vi "Edit a Button--Material.vi"() -> ()   [LabVIEW 2021, in "TSC Button Editor.lvclass"]
doc: "Edit/create buttons based on a few built-in templates.\n\n<b>Code Developed By:</b>\nTechnology Service Corporation\n1983 S Liberty Drive\nBloomington, IN 47403\nPhone: 812 558-7100\nwww.tsc.com/atcs\n\nDeveloper:\nDaniel Coons"
uses:
  TSC Button Editor.lvclass
  TSC Button Editor.lvclass/TSC Button Editor.ctl
  <vilib>/Utility/miscctls.llb/LVPositionTypeDef.ctl
  user32.dll
  Material Theme/Material Theme.lvclass
  Material-Scheme/Material-Scheme.lvclass
panel:
  in  "Tab Control 2":enum32{"Button Format", "Glyphs"}(tab)
  in  "Lock Text in Center?":bool
  in  "update text format":bool
  in  "Boolean Colors":T1={"false color"={"border"=15922170, "fill"=15922170}, "true color"={"border"=14936305, "fill"=14936305}, "click false color"={"border"=14410221, "fill"=14410221}, "click true color"={"border"=14410221, "fill"=14410221}, "hover false color"={"border"=14540516, "fill"=14540516}, "hover true color"={"border"=14540516, "fill"=14540516}}
  in  "Boolean Text Format":T2={"Font:Color"=3563918, "Font:Bold?"=TRUE, "Font:Name"="App Font", "Font:Size"=22}
  in  "Boolean Text":string
  in  "update colors":bool
  in  "Button Size":cluster{"Width":u32, "Height":u32}={"Width"=204, "Height"=48}
  in  "update button size":bool
  in  "Button Text Location":cluster{"Left":i32, "Top":i32}
  in  "update button text location":bool
  in  "edit":bool
  out "Images":T3(array[cluster]) caption="Array"
  in  "Filter":string
  out "images directory":path
  in  "Button Family":u16(ring) items=["(1) Small Button Single Image 24px", "(2) Small Button Text Only", "(3) Large Button Single Image 40px", "(4) Large Button Text Only", "(5) Small Button Multi Image 24px", "(6) Large Button Multi Image 40px", "(7) Floating Action Button (FAB)"]
  in  "Color Level":u16(ring) items=["Primary", "Secondary", "Tertiary", "Error", "Primary Fixed", "Secondary Fixed", "Tertiary Fixed"]
  in  "Theme":u16(ring) items=["Light Theme", "Light Medium Contrast", "Light High Contrast", "Dark Theme", "Dark Medium Contrast", "Dark High Constrast"]
  in  "theme path":path
  in  "Open":bool
  in  "Button Type":u16(ring) items=["elevated--rectangular--icon.ctl", "elevated--rounded--icon.ctl", "filled--rectangular--icon.ctl", "filled--rounded--icon.ctl", "nooutline--rectangular--icon.ctl", "nooutline--rounded--icon.ctl", "outline--rectangular--icon.ctl", "outline--rounded--icon.ctl", "tonal--rectangular--icon.ctl", "tonal--rounded--icon.ctl", "transparent--rectangular--icon.ctl", "transparent--rounded--icon.ctl"]
  in  "Tab Control":enum32{"Button Formatting"}(tab)
  in  "Image Color":u32(colorbox)=3563918
  in  "Button Image":path
  in  "Button Images":T4
  in  "Multiple Colors":T5={"False Color"=3563918, "True Color"=3563918, "True Press"=3563918, "False Press"=3563918}
  out "b":u8
  out "g":u8
  out "r":u8
  out "Color":u32(colorbox)
  in  "Hex Color":u32 max=16777215 format="%06x"
  in  "close":bool
  out "header":bool
  in  "Save":bool
  out "error out":errorcluster
  # "Note: match the size of the replacement image so scaling is correct.\nNormal size: 24x24px, Large size: 40x40px, Icon size: 30x30px\n\nFor other desired sizes, save the control and open it in LabVIEW. Click the Wrench in the tool bar to change to Edit Mode."
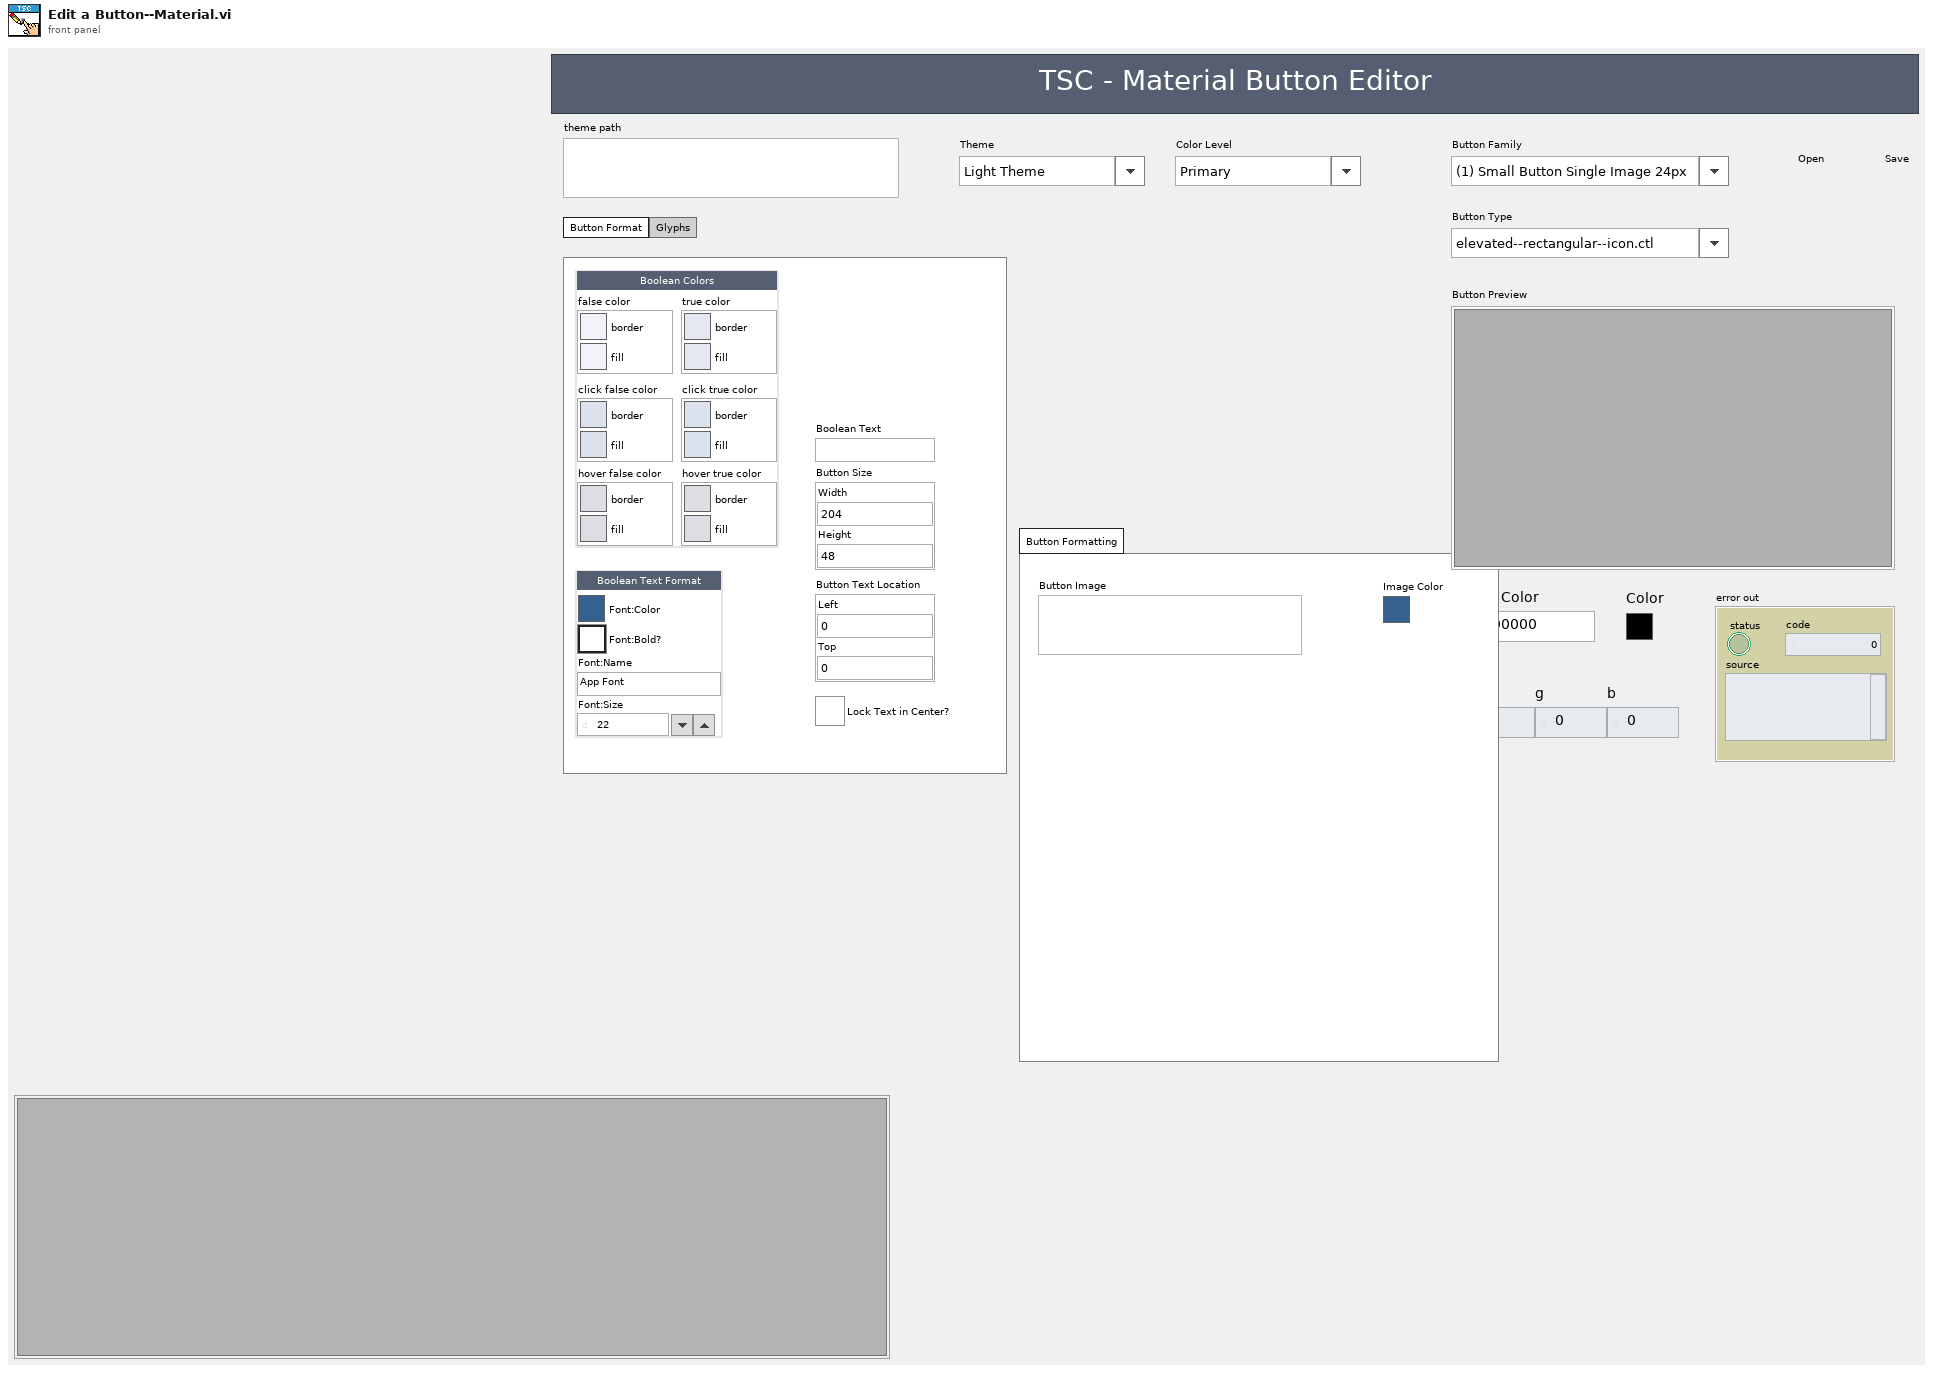
[diagram p1: front panel]
types:
  T1 = cluster{"false color":cluster{"border":u32, "fill":u32}, "true color":cluster{"border":u32, "fill":u32}, "click false color":cluster{"border":u32, "fill":u32}, "click true color":cluster{"border":u32, "fill":u32}, "hover false color":cluster{"border":u32, "fill":u32}, "hover true color":cluster{"border":u32, "fill":u32}}
  T2 = cluster{"Font:Color":u32, "Font:Bold?":bool, "Font:Name":string, "Font:Size":u32}
  T3 = cluster{"2D Picture":picture, "path":path, "image-name":string}[][]
  T4 = cluster{"False Image":path, "True Image":path, "True Press":path, "False Press":path}
  T5 = cluster{"False Color":u32, "True Color":u32, "True Press":u32, "False Press":u32}
  T6 = cluster{"2D Picture":picture, "path":path, "image-name":string}[]
  T7 = typedef "TSC Button Editor.lvclass/User Events.ctl" = cluster{"update colors":refnum<user-event>, "update boolean data":refnum<user-event>, "update image":refnum<user-event>, "update multi image":refnum<user-event>}
  T8 = typedef "LVPositionTypeDef.ctl" = cluster{"Left":i32, "Top":i32}
  T9 = enum32{"invalid VI type", "Standard VI", "Control VI", "Global VI", "Polymorphic VI", "Configuration VI", "SubSystem", "Facade VI", "Method VI", "Statechart Diagram VI"}
  T10 = typedef "LVBoundsTypeDef.ctl" = cluster{"Width":u32, "Height":u32}
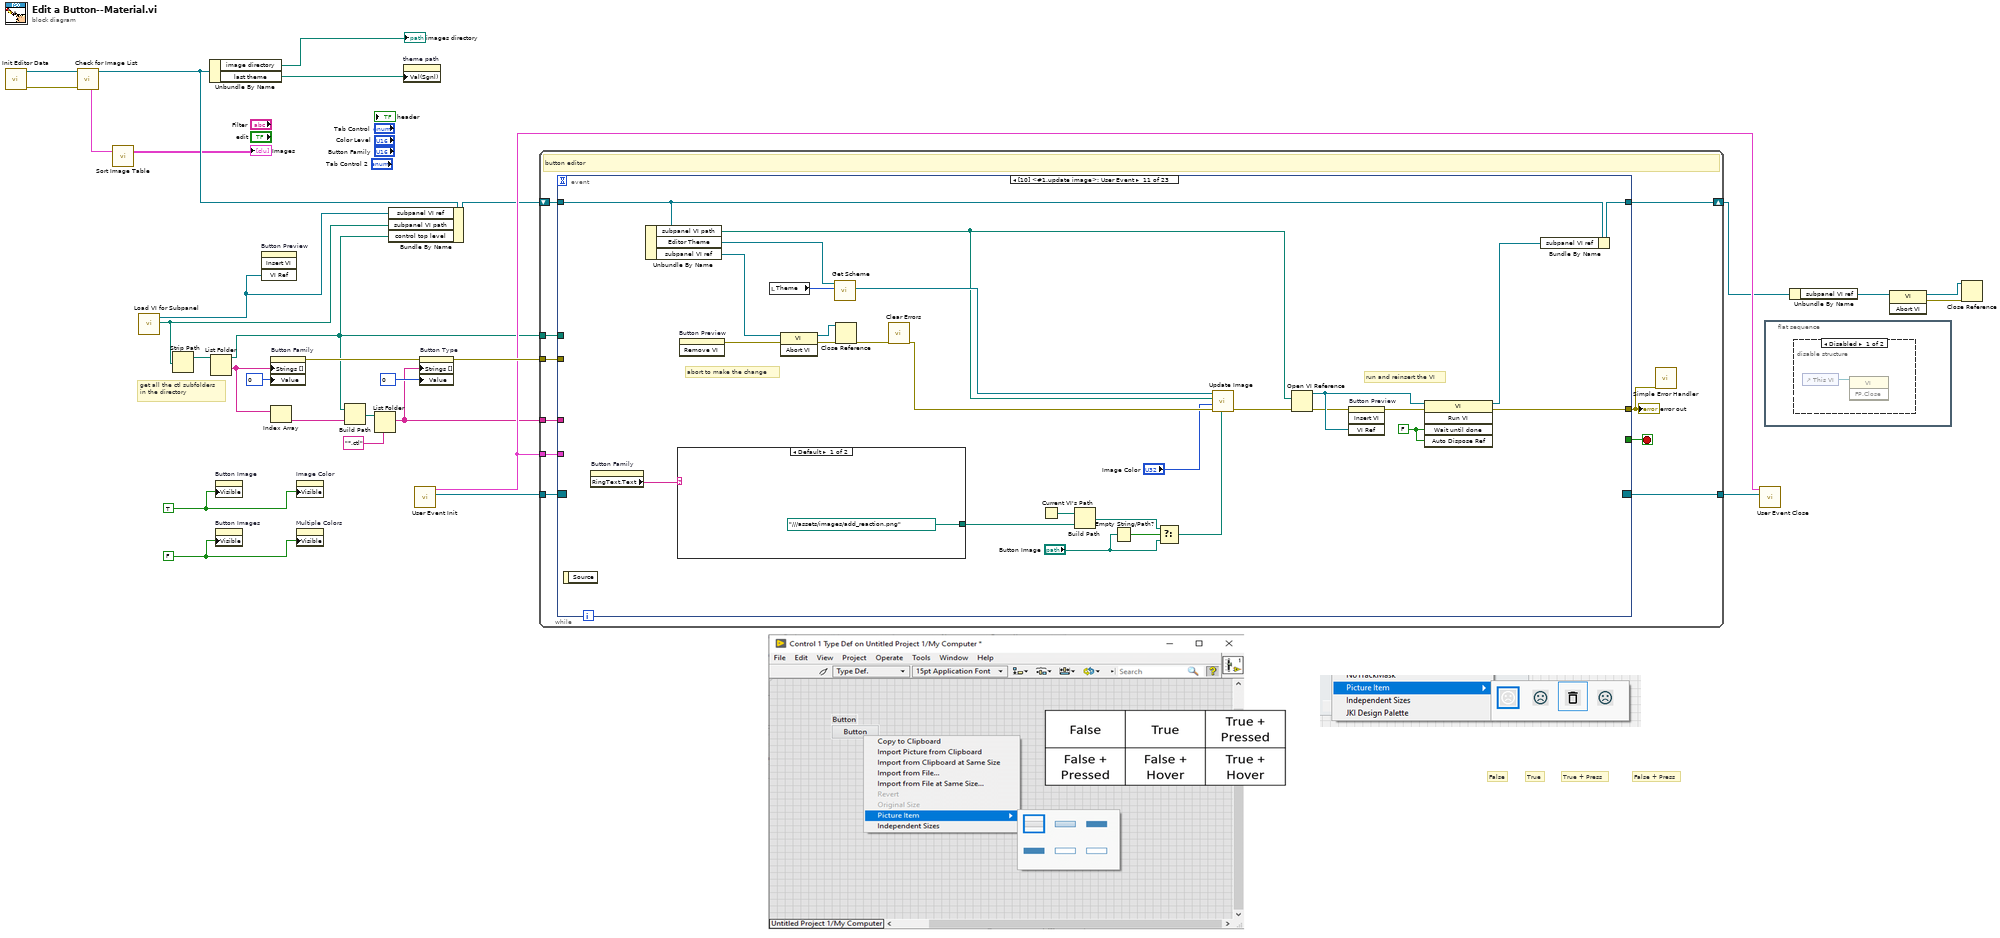
[diagram p0: block diagram]
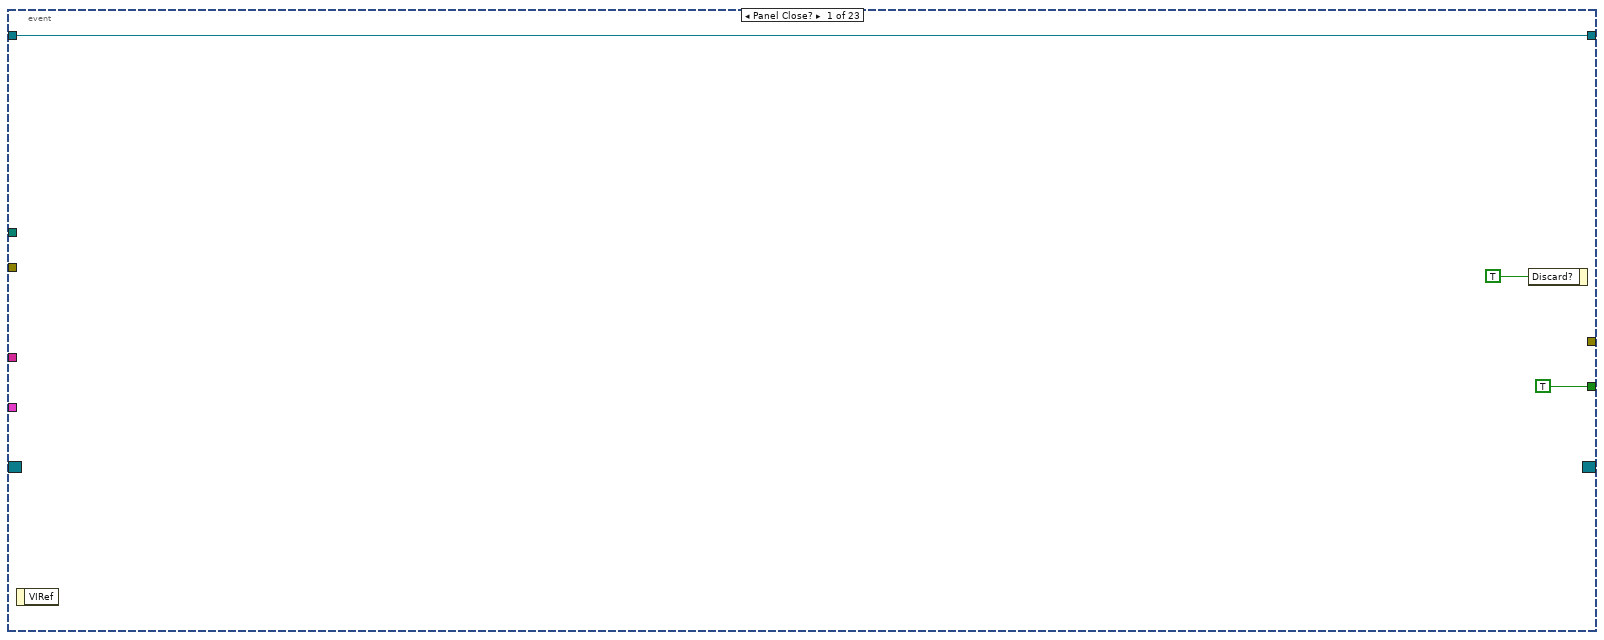
[diagram p3: hidden frame]
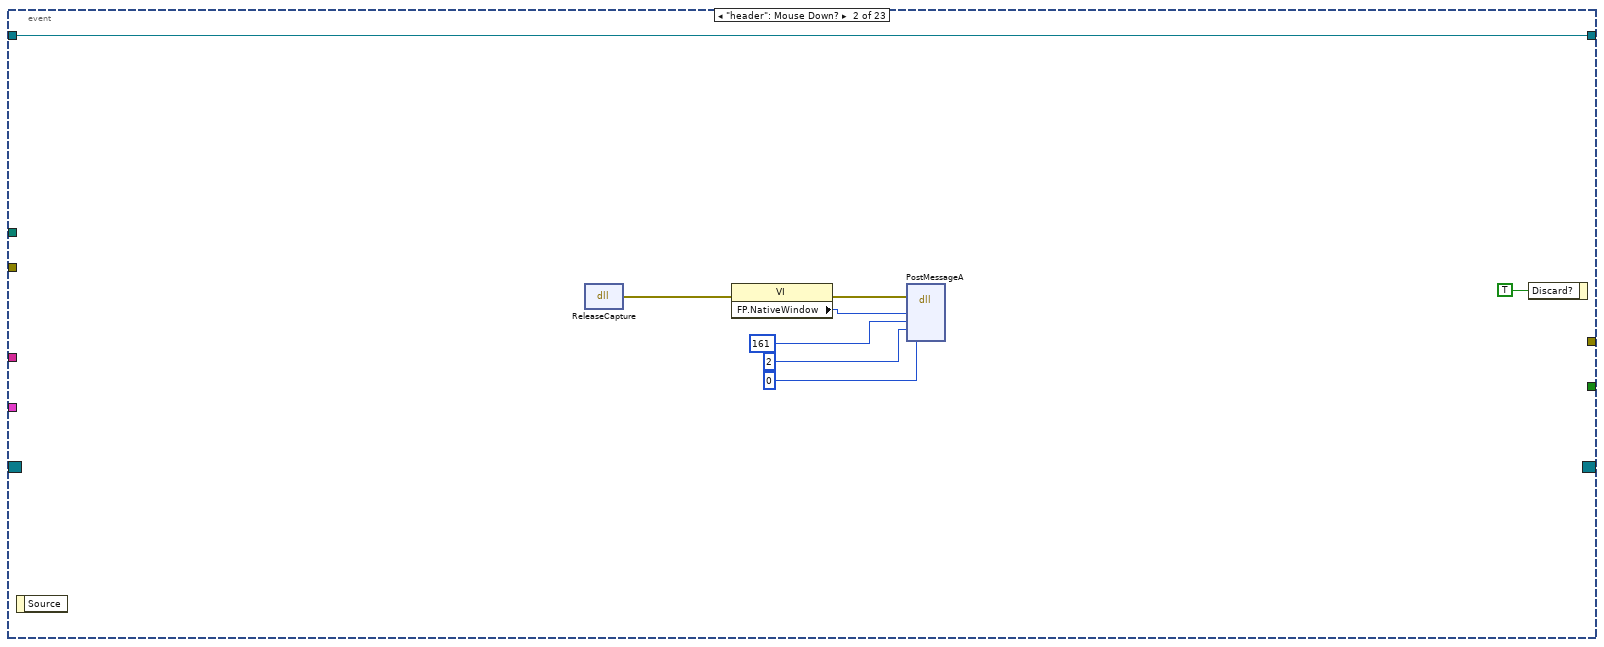
[diagram p4: hidden frame]
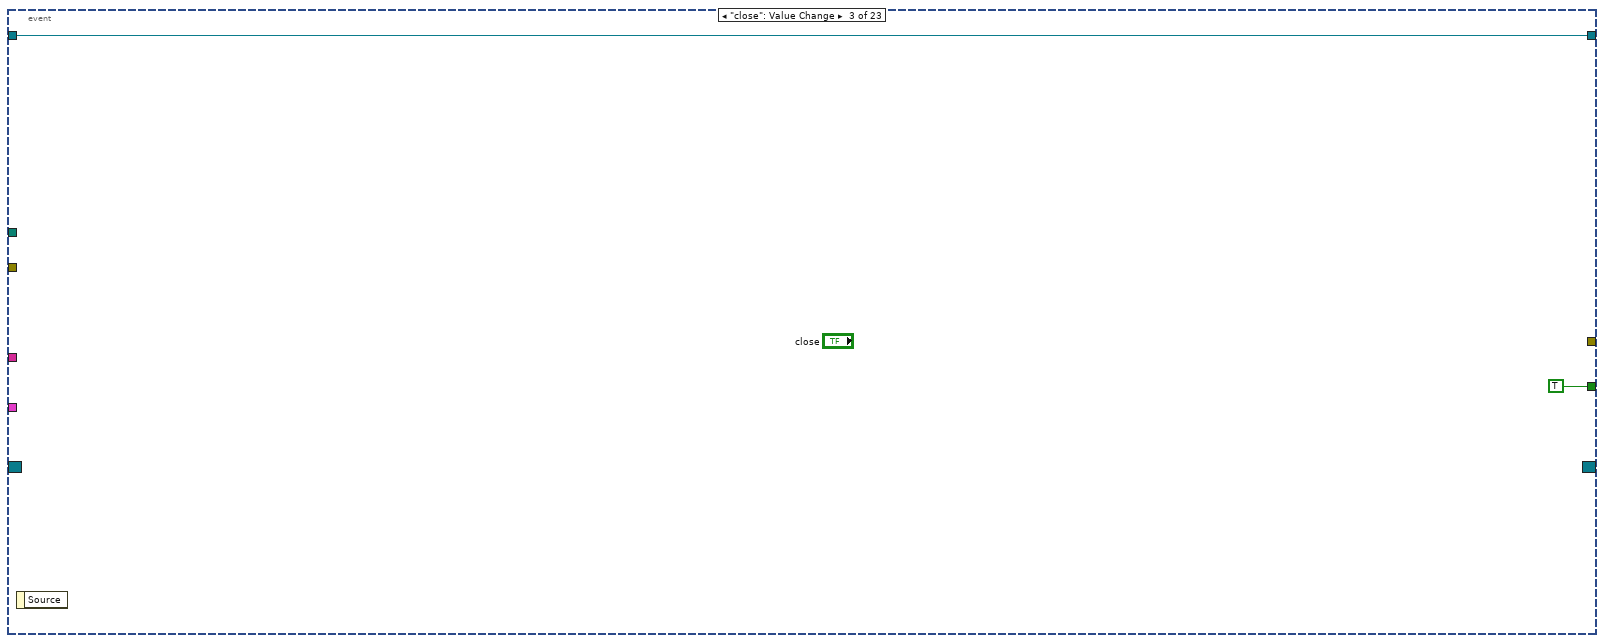
[diagram p5: hidden frame]
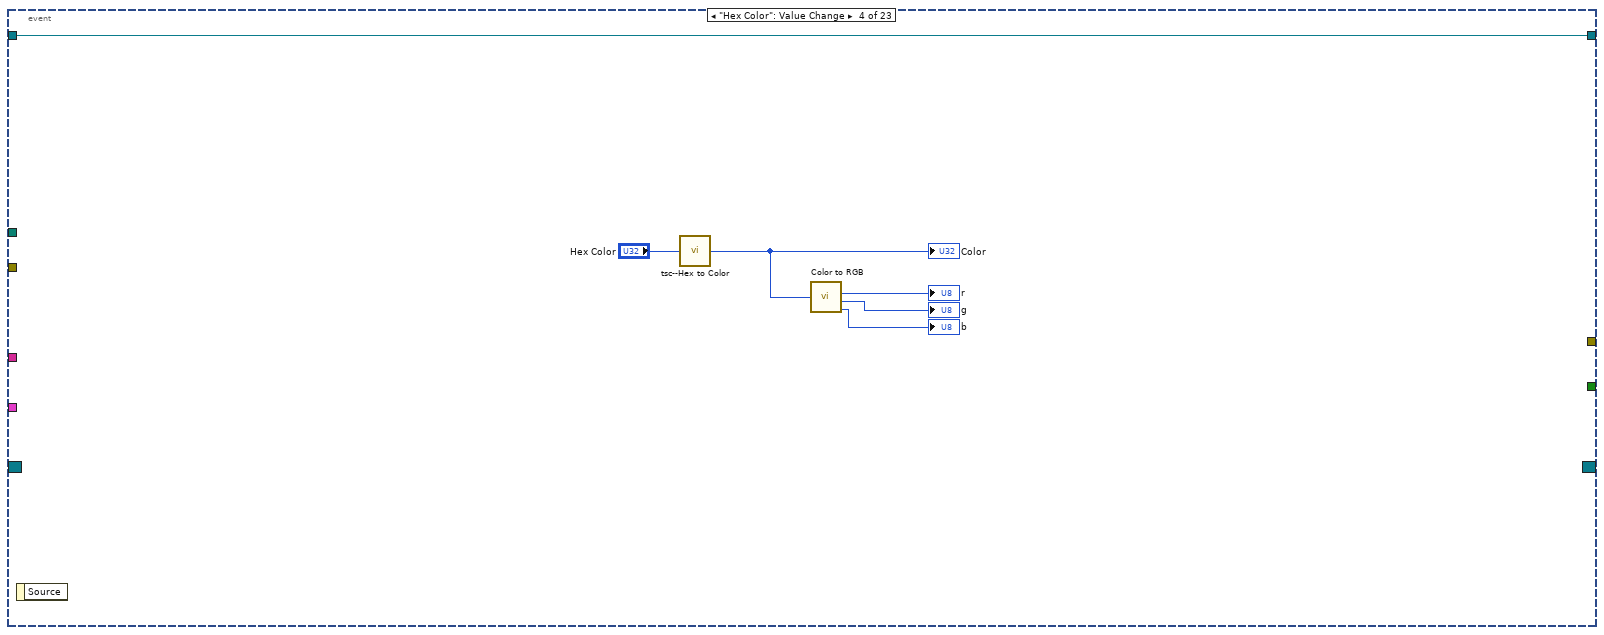
[diagram p6: hidden frame]
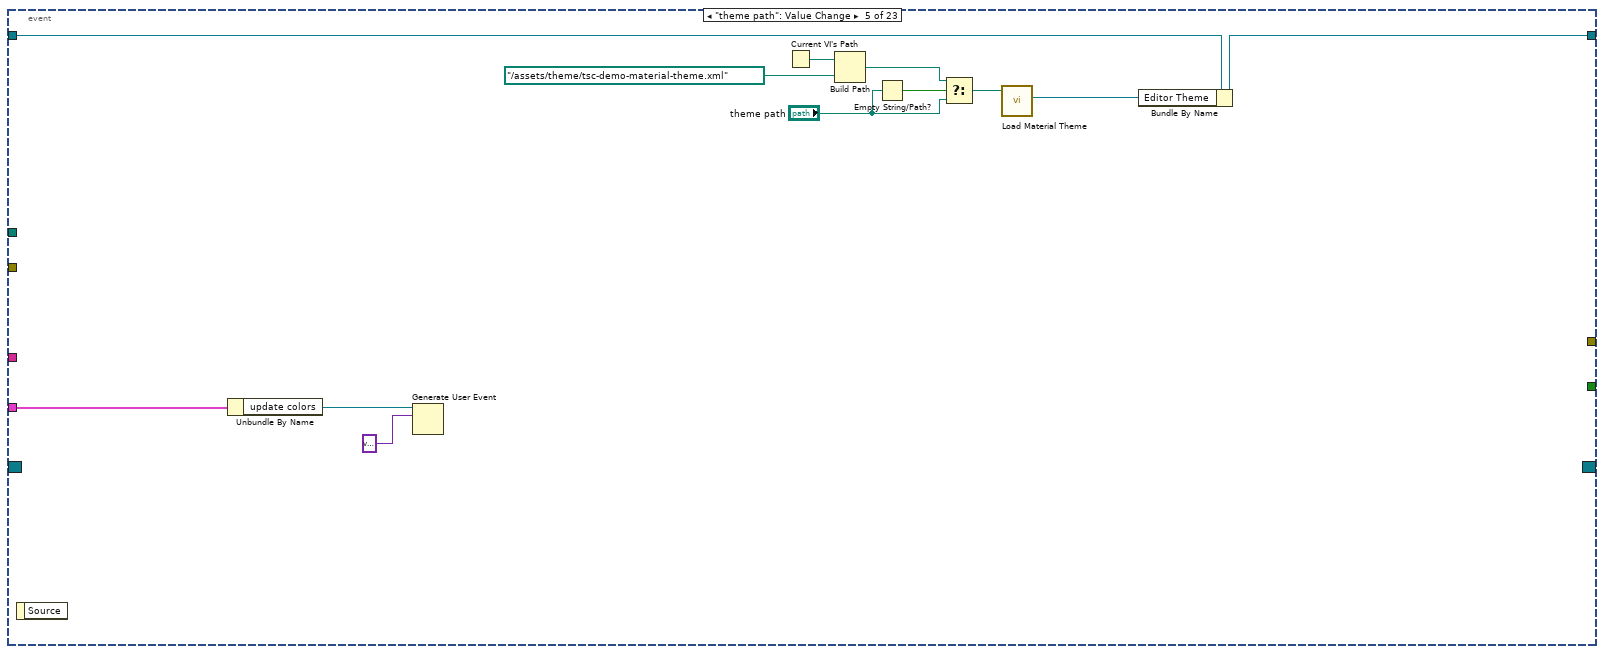
[diagram p7: hidden frame]
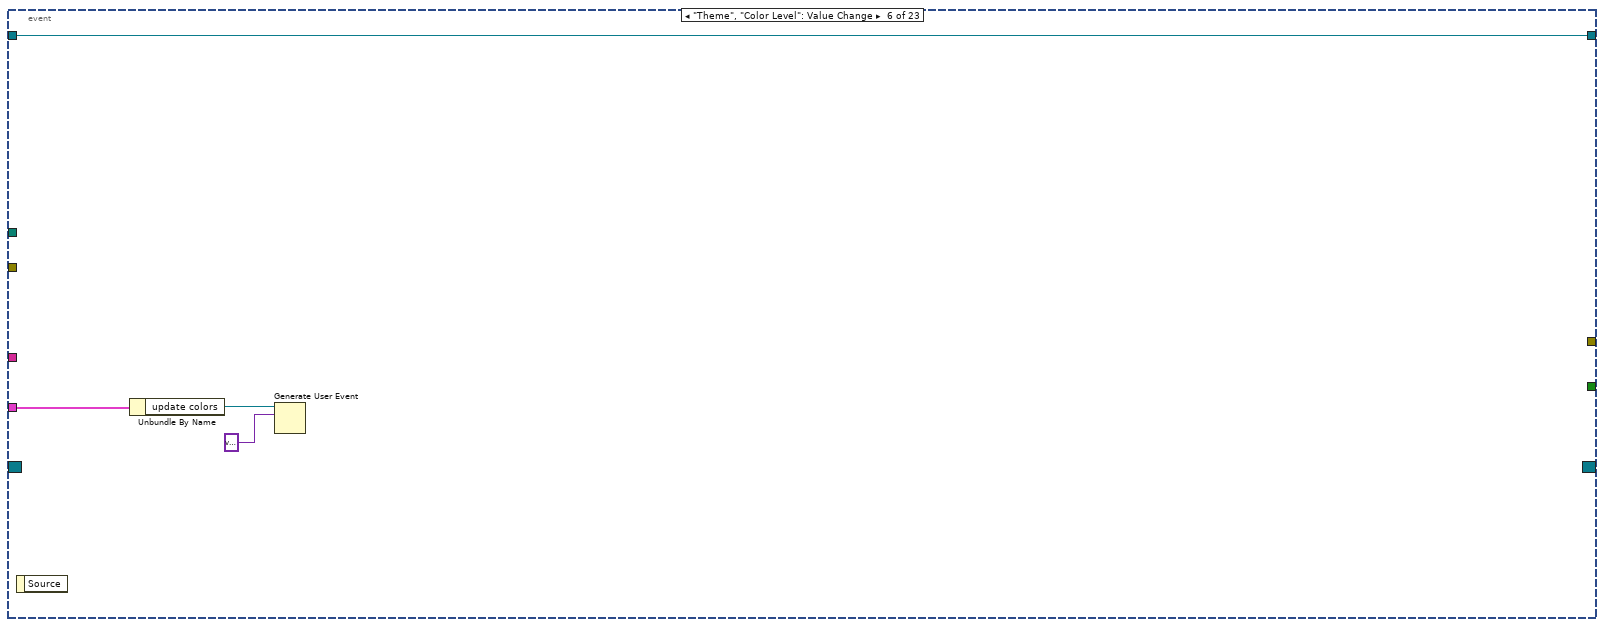
[diagram p8: hidden frame]
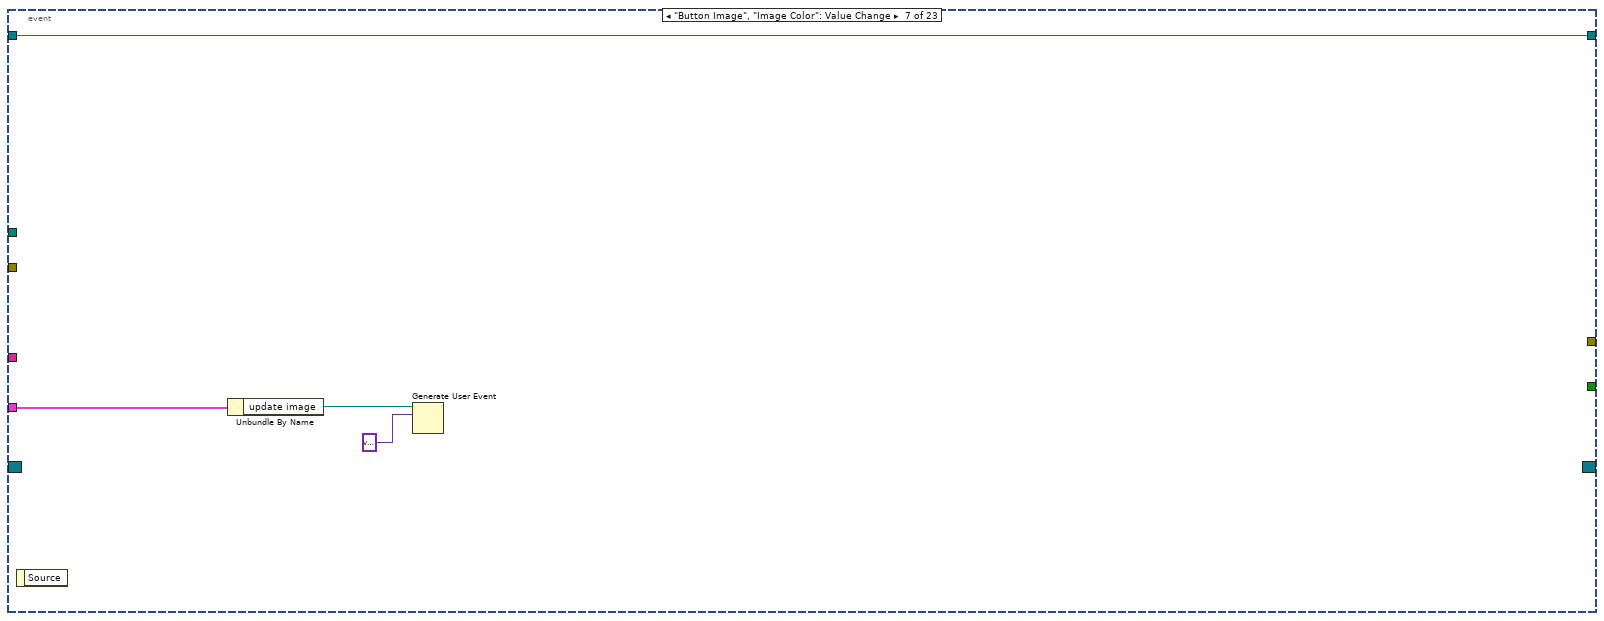
[diagram p9: hidden frame]
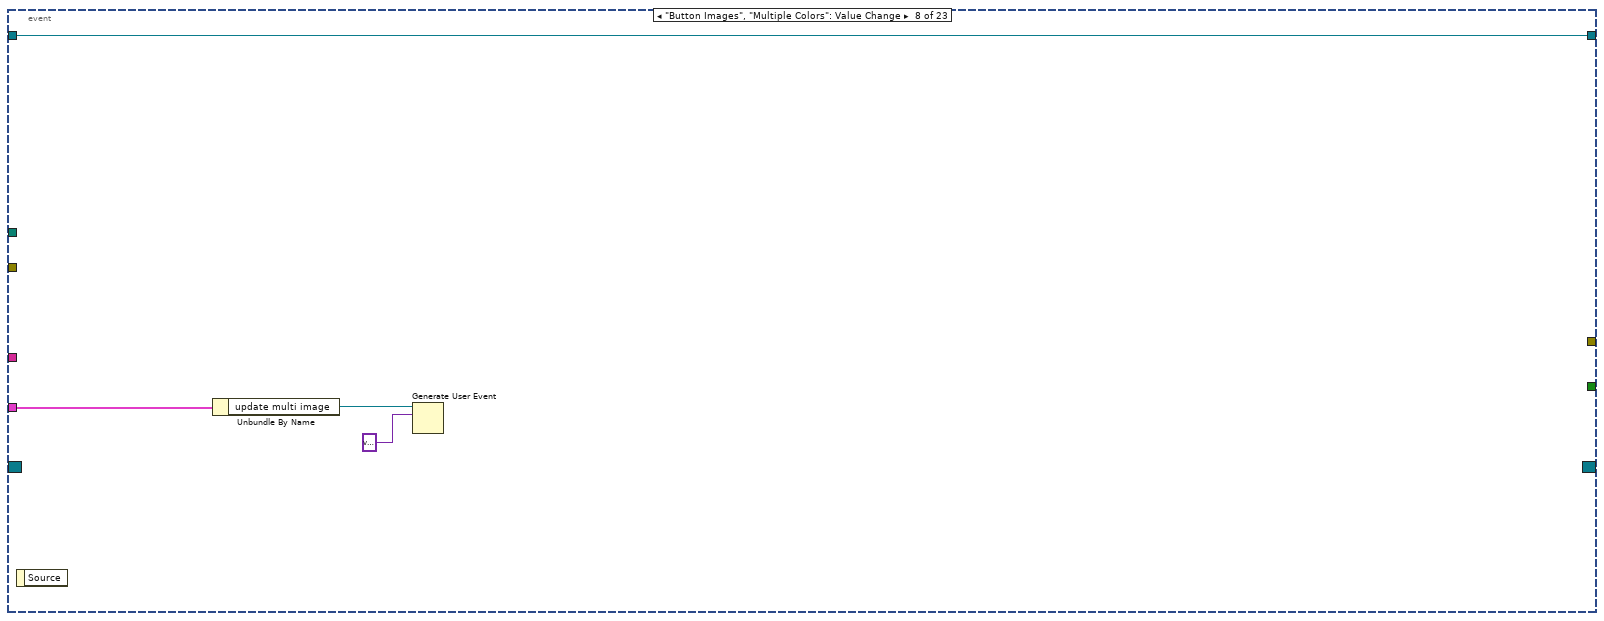
[diagram p10: hidden frame]
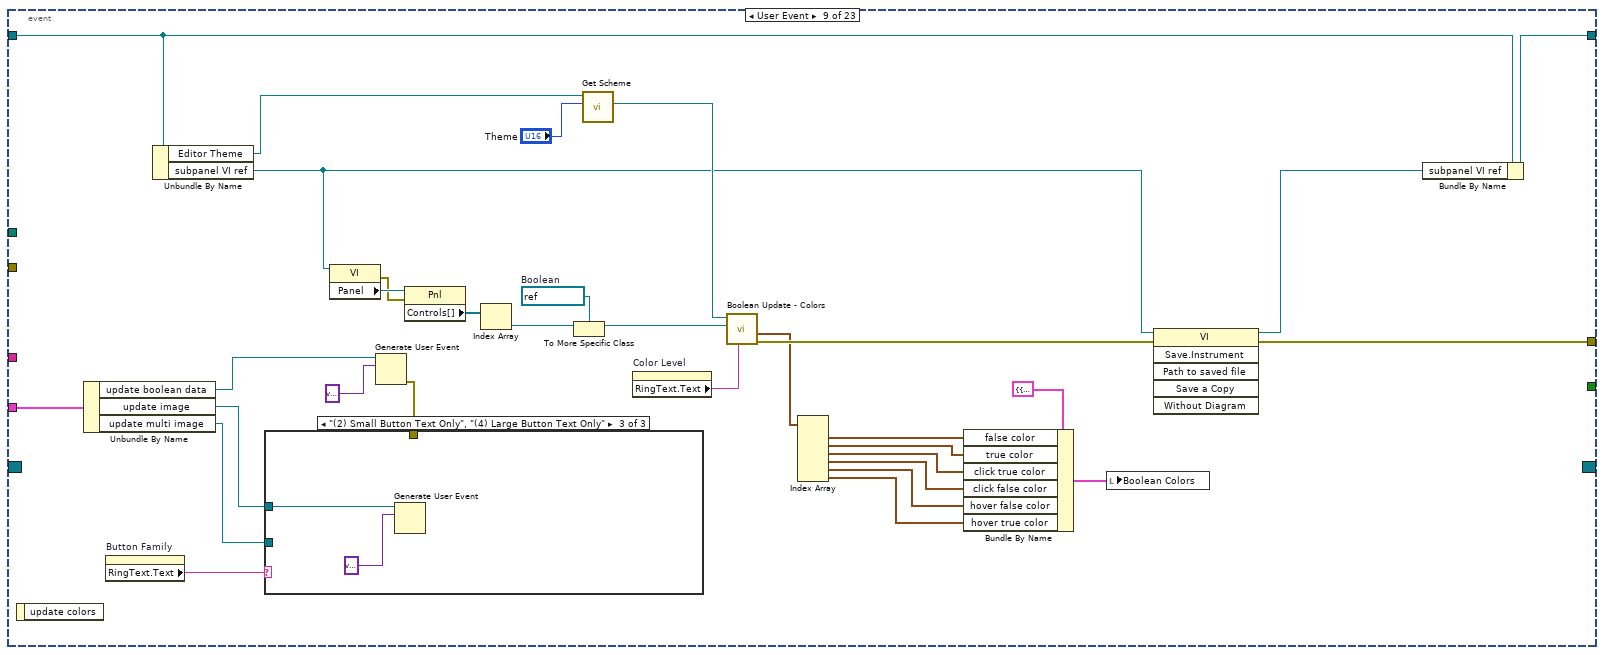
[diagram p11: hidden frame]
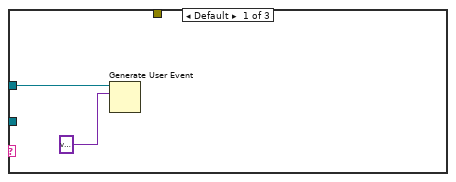
[diagram p12: hidden frame]
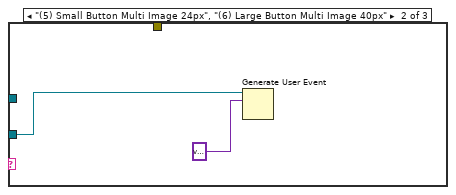
[diagram p13: hidden frame]
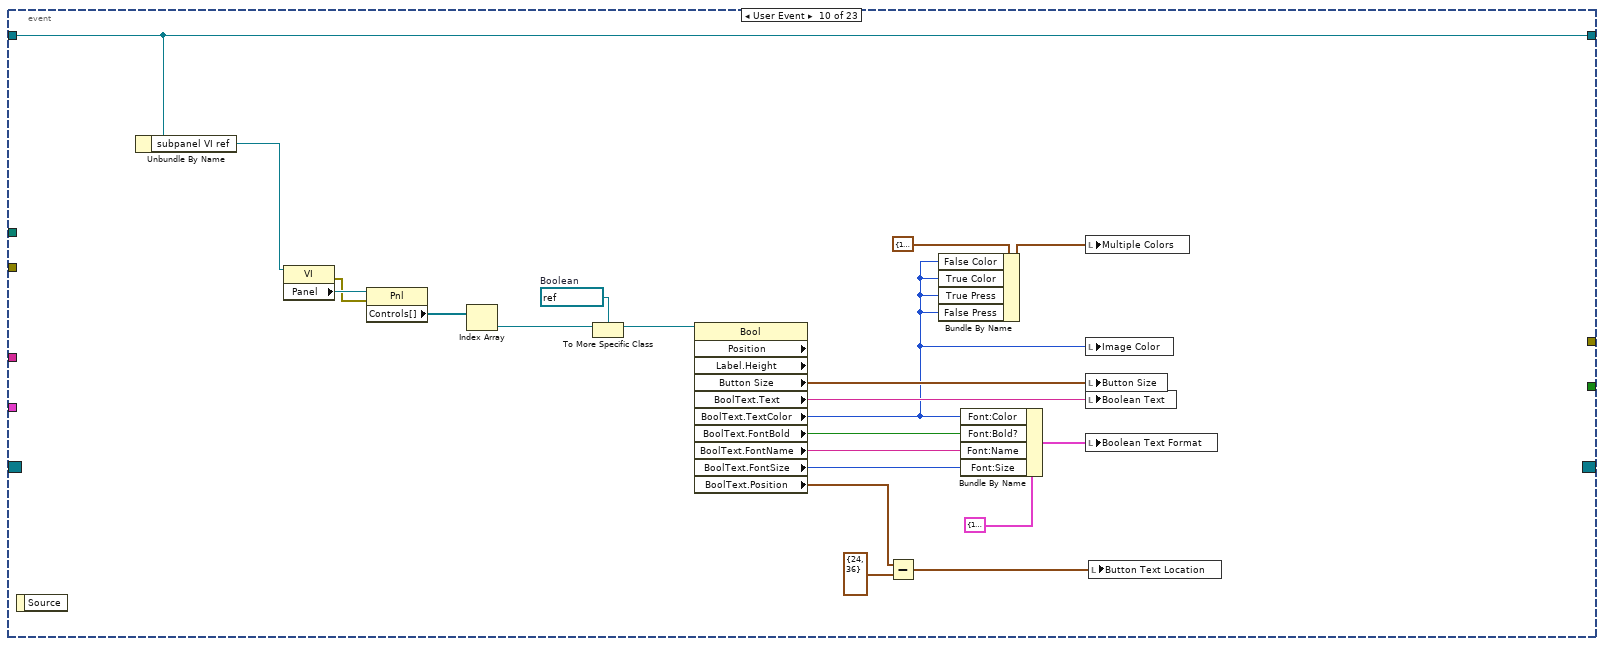
[diagram p14: hidden frame]
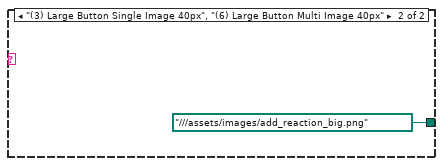
[diagram p15: hidden frame]
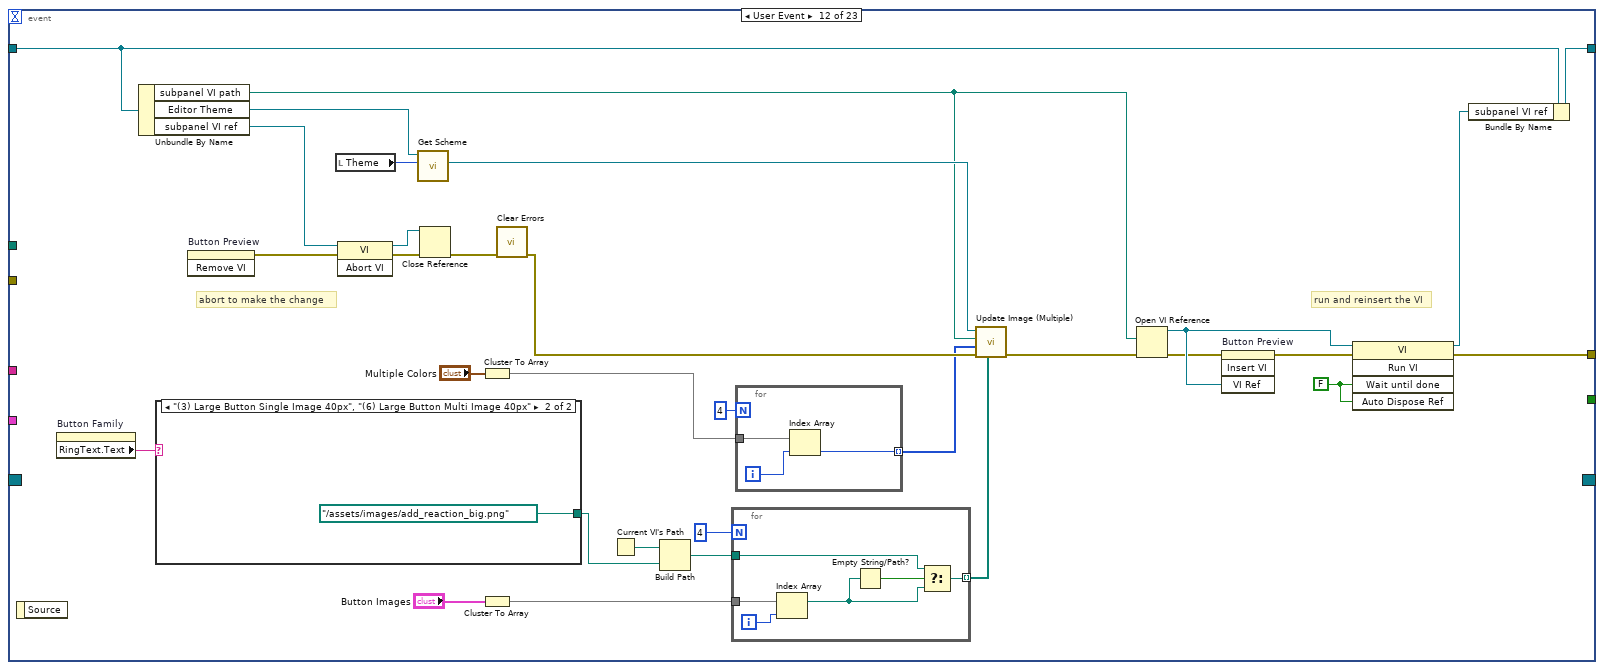
[diagram p16: hidden frame]
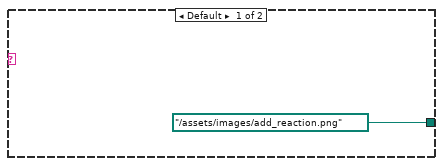
[diagram p17: hidden frame]
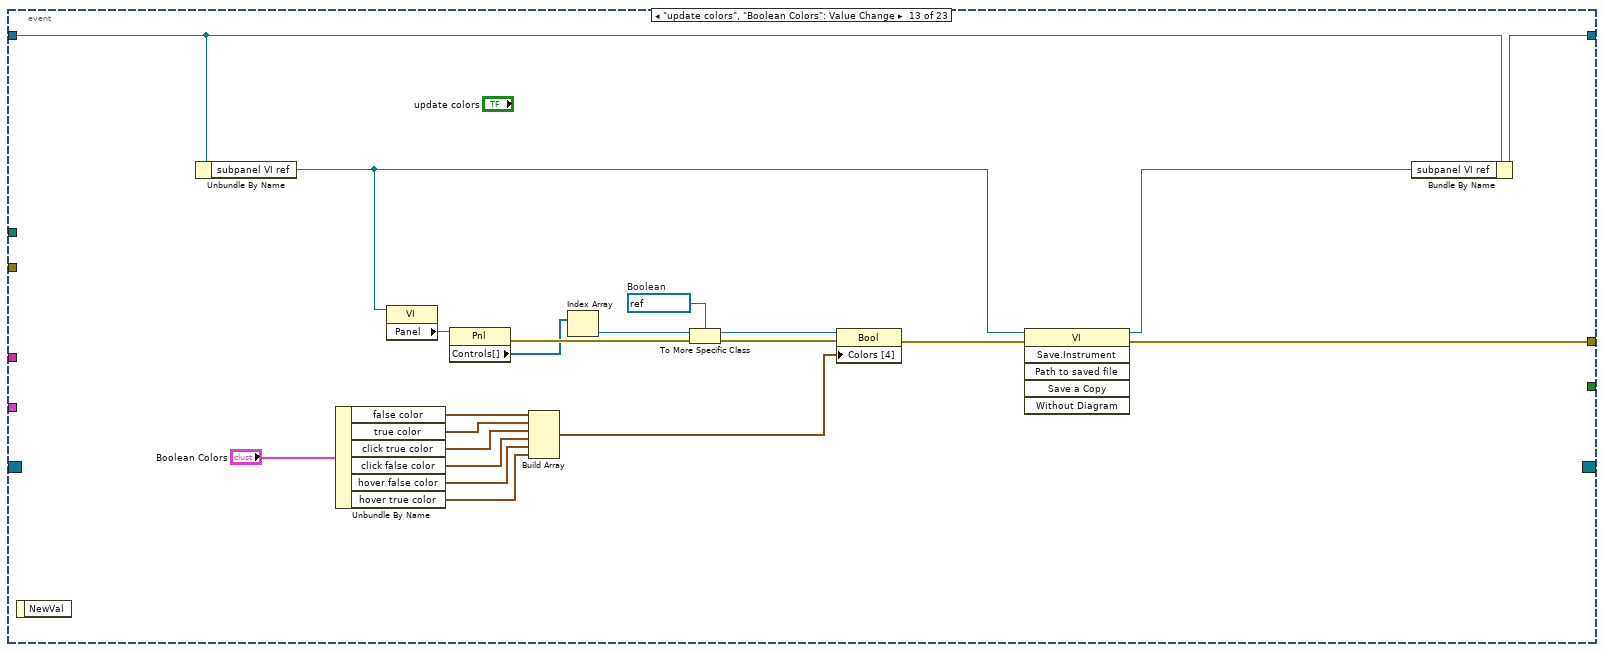
[diagram p18: hidden frame]
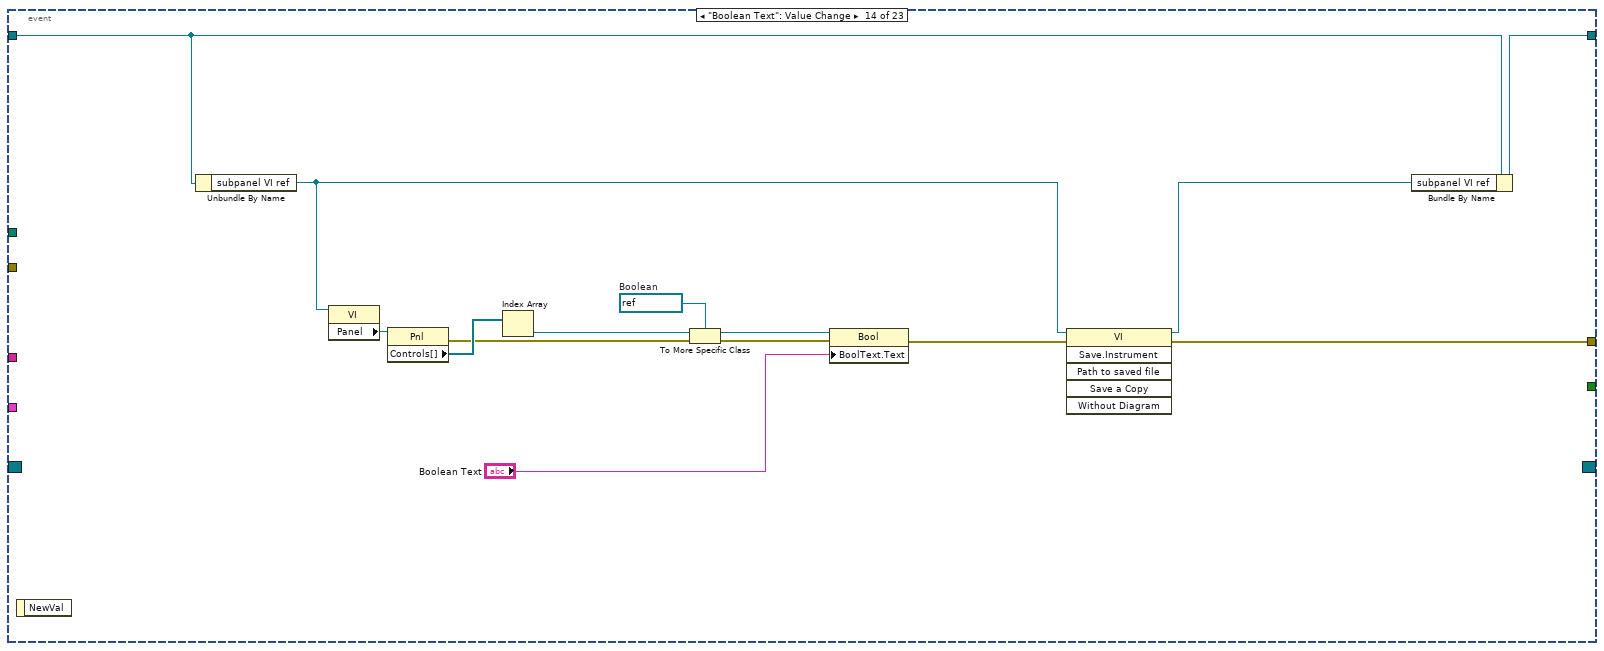
[diagram p19: hidden frame]
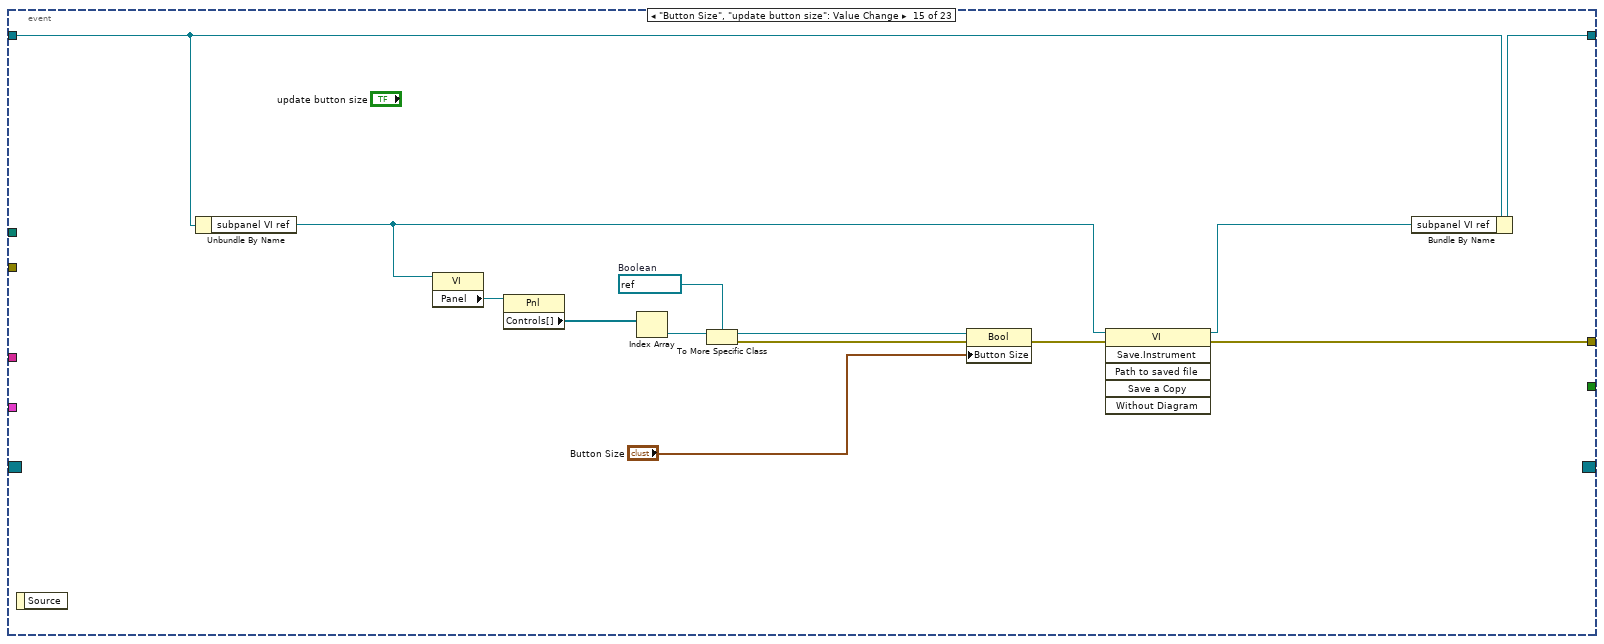
[diagram p20: hidden frame]
diagram:
  w14 = FALSE
  w15 = TRUE
  w17 = u16 0 items=[""] ("Button Type")
  w22 = u16 0 items=[""] ("Button Family")
  # "False + Press"
  # "True + Press"
  # "True"
  # "False"
  # "get all the ctl subfolders\nin the directory"
  n1 = call "Init Editor Data.vi"() -> ("error out"=w1:errorcluster, "TSC Button Editor"=w5:refnum<class "TSC Button Editor.lvclass">)  [unwired: 10 in]
  n2 = call "Check for Image List.vi"("error in"=w1, "TSC Button Editor in"=w5) -> ("TSC Button Editor out"=w4:refnum<class "TSC Button Editor.lvclass">, "Images"=w3:T6)  [unwired: 7 in, 1 out]
  n3 = call "Sort Image Table.vi"("Images in"=w3) -> ("Images out"=→"Images":T3)  [unwired: 2 in]
  n4 = call "Load VI for Subpanel.vi"() -> ("VI Path"=w9:path, "VI out"=w10:refnum<vi>)  [unwired: 10 in]
  n5 = Strip Path(path=w9) -> (stripped path=w27:path)  [unwired: 1 out]
  n6 = Unbundle By Name(w4) -> ("image directory"=→"images directory":path, "last theme"=w13:path)
  n7 = List Folder(path=w27) -> (path out=w8:path, folder names=w21:string[])  [unwired: 3 in, 2 out]
  n8 = property on="Button Image" class="Path"("Visible"=w15) -> ()  [unwired: 2 in, 2 out]
  n9 = property on="Button Images" class="Clust (strict)"("Visible"=w14) -> ()  [unwired: 2 in, 2 out]
  n10 = invoke on="Button Preview" class="SubPnl" method="Insert VI"("VI Ref"=w10) -> ()  [unwired: 3 in, 4 out]
  n11 = property on="Button Family" class="Ring (strict)"("Strings []"=w21, "Value"=w22) -> (error out=w23:errorcluster)  [unwired: 2 in, 1 out]
  n12 = Index Array(array=w21) -> (element=w20:string)  [unwired: 1 in]
  n13 = property on="Image Color" class="ColBox"("Visible"=w15) -> ()  [unwired: 2 in, 2 out]
  n14 = property on="Multiple Colors" class="Clust (strict)"("Visible"=w14) -> ()  [unwired: 2 in, 2 out]
  n15 = Build Path(base path=w8, name or relative path=w20) -> (appended path=w19:path)
  n16 = List Folder(path=w19, pattern="*.ctl") -> (filenames=w16:string[])  [unwired: 2 in, 3 out]
  n17 = Bundle By Name(cluster=w4, "subpanel VI ref"=w10, "subpanel VI path"=w9, "control top level"=w8) -> (w11:refnum<class "TSC Button Editor.lvclass">)
  n18 = property on="theme path" class="Path"("Val(Sgnl)"=w13) -> ()  [unwired: 2 in, 2 out]
  n19 = call "User Event Init.vi"() -> ("Event Registration Refnum"=w26:refnum<event-registration>, "user events"=w24:T7)  [unwired: 10 in]
  n20 = property on="Button Type" class="Ring (strict)"(error in=w23, "Strings []"=w16, "Value"=w17) -> (error out=w28:errorcluster)  [unwired: 1 in, 1 out]
  n21 = while {
    tunnel: w28 -> [w39]
    tunnel: w26 -> [w38]
    tunnel: [w37] -> w25
    tunnel: w24 -> [w36]
    tunnel: w16 -> [w35]
    tunnel: w8 -> [w33]
    shift-right: [w31] -> w7
    shift-left: w11 -> [w32]
    stop <- w40 stop-if-true
    # "button editor"
    n22 = event shown="[10] <#1.update image>: User Event" {
      selector: w38 -> [_ _ _ _ _ _ _ _ _ _ _ _ _ _ _ _ _ _ _ _ _ _ _]
      dyn-events: [_ _ _ _ _ _ _ _ _ _ _ _ _ _ _ _ _ _ _ _ _ _ _] -> w37
      timeout: _ -> [_ _ _ _ _ _ _ _ _ _ _ _ _ _ _ _ _ _ _ _ _ _ _]
      tunnel: [TRUE _ TRUE _ _ _ _ _ _ _ _ _ _ _ _ _ _ _ _ _ _ _ _] -> w40
      tunnel: [_ _ _ _ _ _ _ _ w110 _ w156 w190 w231 w243 w253 w262 w279 w294 w314 w344 w401 _ w430] -> w34
      tunnel: w39 -> [_ _ _ _ _ _ _ _ _ _ _ _ _ _ _ _ _ _ _ _ _ _ _]
      tunnel: w36 -> [_ _ _ _ w71 w75 w79 w83 w111 _ _ _ _ _ _ _ _ _ _ _ w390 _ _]
      tunnel: w35 -> [_ _ _ _ _ _ _ _ _ _ _ _ _ _ _ _ _ _ _ _ _ _ _]
      tunnel: w33 -> [_ _ _ _ _ _ _ _ _ _ _ _ _ _ _ _ _ _ _ _ _ _ _]
      tunnel: w32 -> [w41 w44 w52 w54 w62 w72 w76 w80 w88 w123 w145 w174 w217 w236 w250 w265 w277 w292 w310 w342 w380 w414 w428]
      tunnel: [w41 w44 w52 w54 w61 w72 w76 w80 w86 w123 w144 w173 w216 w235 w249 w264 w278 w293 w310 w342 w379 w414 w428] -> w31
      event Panel Close? {
        n23 = event-data() -> ()  [unwired: 1 in, 1 out]
        n24 = event-data("Discard?"=TRUE) -> ()  [unwired: 1 in, 1 out]
      }
      event "header": Mouse Down? {
        n25 = event-data() -> ()  [unwired: 1 in, 1 out]
        n26 = dll-call lib="user32.dll" fn="ReleaseCapture"() -> (error out=w47:errorcluster)  [unwired: 4 in, 1 out]
        n27 = property class="VI"(error in=w47) -> (error out=w46:errorcluster, "FP.NativeWindow"=w45:u64)  [unwired: 1 in, 1 out]
        n28 = dll-call lib="user32.dll" fn="PostMessageA"(error in=w46, "hWnd"=w45, "Msg"=161, "wParam"=2, "lParam"=0) -> ()  [unwired: 7 in, 2 out]
        n29 = event-data("Discard?"=TRUE) -> ()  [unwired: 1 in, 1 out]
      }
      event "close": Value Change {
        n30 = event-data() -> ()  [unwired: 1 in, 1 out]
      }
      event "Hex Color": Value Change {
        n31 = event-data() -> ()  [unwired: 1 in, 1 out]
        n32 = call "tsc--Hex to Color.vi"("Hex String"="Hex Color") -> ("Color Box"=w55:u32)  [unwired: 4 in]
        "Color" <- w55
        n33 = call <vilib>:"Color to RGB.vi"("Color"=w55) -> ("R"=→"r":u8, "G"=→"g":u8, "B"=→"b":u8)  [unwired: 1 out]
      }
      event "theme path": Value Change {
        n34 = event-data() -> ()  [unwired: 1 in, 1 out]
        n35 = Unbundle By Name(w71) -> ("update colors"=w69:refnum<user-event>)
        n36 = Generate User Event(user event=w69, event data cluster=variant ("event data")) -> ()  [unwired: 2 in, 2 out]
        n37 = Current VI's Path() -> (path=w67:path)
        n38 = Build Path(base path=w67, name or relative path=path "../assets/theme/tsc-demo-material-theme.xml") -> (appended path=w65:path)
        n39 = Empty String/Path?(string/path="theme path") -> (empty?=w68:bool)
        n40 = Select(t=w65, s=w68, f="theme path") -> (s? t:f=w63:path)
        n41 = call "Load Material Theme.vi"("file path (use dialog)"=w63) -> ("Theme"=w60:refnum<class "Material Theme.lvclass">)  [unwired: 9 in, 1 out]
        n42 = Bundle By Name(cluster=w62, "Editor Theme"=w60) -> (w61:refnum<class "TSC Button Editor.lvclass">)
      }
      event "Theme", "Color Level": Value Change {
        n43 = event-data() -> ()  [unwired: 1 in, 1 out]
        n44 = Unbundle By Name(w75) -> ("update colors"=w73:refnum<user-event>)
        n45 = Generate User Event(user event=w73, event data cluster=variant ("event data")) -> ()  [unwired: 2 in, 2 out]
      }
      event "Button Image", "Image Color": Value Change {
        n46 = event-data() -> ()  [unwired: 1 in, 1 out]
        n47 = Unbundle By Name(w79) -> ("update image"=w77:refnum<user-event>)
        n48 = Generate User Event(user event=w77, event data cluster=variant ("event data")) -> ()  [unwired: 2 in, 2 out]
      }
      event "Button Images", "Multiple Colors": Value Change {
        n49 = event-data() -> ()  [unwired: 1 in, 1 out]
        n50 = Unbundle By Name(w83) -> ("update multi image"=w81:refnum<user-event>)
        n51 = Generate User Event(user event=w81, event data cluster=variant ("event data")) -> ()  [unwired: 2 in, 2 out]
      }
      event User Event {
        w100 = refnum<vi> refnum  # Boolean
        n52 = event-data() -> ()  [unwired: 1 in, 1 out]
        n53 = Unbundle By Name(w111) -> ("update boolean data"=w113:refnum<user-event>, "update image"=w107:refnum<user-event>, "update multi image"=w108:refnum<user-event>)
        n54 = property on="Button Family" class="Ring (strict)"() -> ("RingText.Text"=w109:string)  [unwired: 2 in, 2 out]
        n55 = Unbundle By Name(w88) -> ("Editor Theme"=w84:refnum<class "Material Theme.lvclass">, "subpanel VI ref"=w87:refnum<vi>)
        n56 = property class="VI"(reference=w87) -> (error out=w102:errorcluster, "Panel"=w105:refnum<vi>)  [unwired: 1 in, 1 out]
        n57 = Generate User Event(user event=w113, event data cluster=variant ("event data")) -> (error out=w106:errorcluster)  [unwired: 2 in, 1 out]
        n58 = case shown="\"(2) Small Button Text Only\", \"(4) Large Button Text Only\"" w109 {
          tunnel: w108 -> [_ w118 _]
          tunnel: w107 -> [w116 _ w120]
          tunnel: w106 -> [_ _ _]
          frame Default {
            n59 = Generate User Event(user event=w116, event data cluster=variant ("event data")) -> ()  [unwired: 2 in, 2 out]
          }
          frame "(5) Small Button Multi Image 24px", "(6) Large Button Multi Image 40px" {
            n60 = Generate User Event(user event=w118, event data cluster=variant ("event data")) -> ()  [unwired: 2 in, 2 out]
          }
          frame "(2) Small Button Text Only", "(4) Large Button Text Only" {
            n61 = Generate User Event(user event=w120, event data cluster=variant ("event data")) -> ()  [unwired: 2 in, 2 out]
          }
        }
        n62 = property class="Pnl"(reference=w105, error in=w102) -> ("Controls[]"=w104:refnum<vi>[])  [unwired: 2 out]
        n63 = Index Array(array=w104) -> (element=w103:refnum<vi>)  [unwired: 1 in]
        n64 = To More Specific Class(target class=w100, reference=w103) -> (specific class reference=w101:refnum<vi>)  [unwired: 1 in, 1 out]
        n65 = call "Get Scheme.vi"("Theme"="Theme", "Material Theme in"=w84) -> ("Material-Scheme"=w115:refnum<class "Material-Scheme.lvclass">)  [unwired: 7 in, 2 out]
        n66 = property on="Color Level" class="Ring (strict)"() -> ("RingText.Text"=w91:string)  [unwired: 2 in, 2 out]
        n67 = call "Boolean Update - Colors.vi"("control-level"=w91, "Bool Refnum"=w101, "Material-Scheme in"=w115) -> ("error out"=w99:errorcluster, "Array"=w98:cluster{"bg":u32, "fg":u32}[])  [unwired: 5 in, 2 out]
        n68 = Index Array(array=w98) -> (element #1=w96:cluster{"bg":u32, "fg":u32}, element #2=w95:cluster{"bg":u32, "fg":u32}, element #3=w89:cluster{"bg":u32, "fg":u32}, element #4=w90:cluster{"bg":u32, "fg":u32}, element #5=w94:cluster{"bg":u32, "fg":u32}, element #6=w93:cluster{"bg":u32, "fg":u32})  [unwired: 6 in]
        n69 = Bundle By Name(cluster=T1 {"false color"={"border"=15922170, "fill"=15922170}, "true color"={"border"=14936305, "fill"=14936305}, "click false color"={"border"=14410221, "fill"=14410221}, "click true color"={"border"=14410221, "fill"=14410221}, "hover false color"={"border"=14540516, "fill"=14540516}, "hover true color"={"border"=14540516, "fill"=14540516}} ("Boolean Colors"), "false color"=w96, "true color"=w95, "click true color"=w89, "click false color"=w90, "hover false color"=w94, "hover true color"=w93) -> (w92:T1)
        n70 = local write "Boolean Colors"(w92) -> ()
        n71 = invoke class="VI" method="Save.Instrument"(reference=w87, error in=w99) -> (reference out=w85:refnum<vi>, error out=w110:errorcluster)  [unwired: 4 in, 4 out]
        n72 = Bundle By Name(cluster=w88, "subpanel VI ref"=w85) -> (w86:refnum<class "TSC Button Editor.lvclass">)
      }
      event User Event {
        w138 = refnum<vi> refnum  # Boolean
        n73 = event-data() -> ()  [unwired: 1 in, 1 out]
        n74 = Unbundle By Name(w123) -> ("subpanel VI ref"=w122:refnum<vi>)
        n75 = property class="VI"(reference=w122) -> (error out=w139:errorcluster, "Panel"=w142:refnum<vi>)  [unwired: 1 in, 1 out]
        n76 = property class="Pnl"(reference=w142, error in=w139) -> ("Controls[]"=w141:refnum<vi>[])  [unwired: 2 out]
        n77 = Index Array(array=w141) -> (element=w140:refnum<vi>)  [unwired: 1 in]
        n78 = To More Specific Class(target class=w138, reference=w140) -> (specific class reference=w137:refnum<vi>)  [unwired: 1 in, 1 out]
        n79 = property class="Bool" props=["Position", "Label", "Height", "Button Size", "BoolText", "Text", "BoolText", "TextColor", "BoolText", "FontBold", "BoolText", "FontName", "BoolText", "FontSize", "BoolText", "Position"](reference=w137) -> ("Button Size"=w136:T10, "BoolText.Text"=w134:string, "BoolText.TextColor"=w127:u32, "BoolText.FontBold"=w133:bool, "BoolText.FontName"=w132:string, "BoolText.FontSize"=w131:u32, "BoolText.Position"=w126:T8)  [unwired: 1 in, 4 out]
        n80 = Subtract(x=w126, y=cluster{"Left":i32, "Top":i32} {"Left"=24, "Top"=36}) -> (x-y=w124:T8)
        n81 = Bundle By Name(cluster=T5 {"False Color"=16777215, "True Color"=16777215, "True Press"=16777215, "False Press"=16777215} ("Multiple Colors"), "False Color"=w127, "True Color"=w127, "True Press"=w127, "False Press"=w127) -> (w128:T5)
        n82 = Bundle By Name(cluster=T2 {"Font:Color"=13140, "Font:Bold?"=TRUE, "Font:Name"="App Font", "Font:Size"=22} ("Boolean Text Format"), "Font:Color"=w127, "Font:Bold?"=w133, "Font:Name"=w132, "Font:Size"=w131) -> (w130:T2)
        n83 = local write "Multiple Colors"(w128) -> ()
        n84 = local write "Image Color"(w127) -> ()
        n85 = local write "Button Size"(w136) -> ()
        n86 = local write "Boolean Text"(w134) -> ()
        n87 = local write "Boolean Text Format"(w130) -> ()
        n88 = local write "Button Text Location"(w124) -> ()
      }
      event User Event {
        w168 = FALSE ("Wait Until Done")
        # "run and reinsert the VI"
        # "abort to make the change"
        n89 = event-data() -> ()  [unwired: 1 in, 1 out]
        n90 = property on="Button Family" class="Ring (strict)"() -> ("RingText.Text"=w150:string)  [unwired: 2 in, 2 out]
        n91 = Unbundle By Name(w145) -> ("subpanel VI path"=w146:path, "Editor Theme"=w147:refnum<class "Material Theme.lvclass">, "subpanel VI ref"=w148:refnum<vi>)
        n92 = case shown="Default" w150 {
          tunnel: [path "../../../assets/images/add_reaction.png" path "../../../assets/images/add_reaction_big.png"] -> w149
          frame Default {
          }
          frame "(3) Large Button Single Image 40px", "(6) Large Button Multi Image 40px" {
          }
        }
        n93 = invoke on="Button Preview" class="SubPnl" method="Remove VI"() -> (error out=w161:errorcluster)  [unwired: 3 in, 2 out]
        n94 = local read "Theme"() -> (w167:u16)
        n95 = invoke class="VI" method="Abort VI"(reference=w148, error in=w161) -> (reference out=w165:refnum<vi>, error out=w169:errorcluster)  [unwired: 1 in, 1 out]
        n96 = call "Get Scheme.vi"("Theme"=w167, "Material Theme in"=w147) -> ("Material-Scheme"=w162:refnum<class "Material-Scheme.lvclass">)  [unwired: 7 in, 2 out]
        n97 = Close Reference(reference=w165, error in (no error)=w169) -> (error out=w166:errorcluster)
        n98 = call <vilib>:"Clear Errors.vi"("error in (no error)"=w166) -> ("error out"=w164:errorcluster)  [unwired: 5 in, 1 out]
        n99 = Current VI's Path() -> (path=w153:path)
        n100 = Build Path(base path=w153, name or relative path=w149) -> (appended path=w152:path)
        n101 = Empty String/Path?(string/path="Button Image") -> (empty?=w155:bool)
        n102 = Select(t=w152, s=w155, f="Button Image") -> (s? t:f=w151:path)
        n103 = call "Update Image.vi"("Replace Image"=w151, "error in"=w164, "New Color"="Image Color", "New Control"=w146, "Material-Scheme.lvclass"=w162) -> ("error out"=w163:errorcluster)  [unwired: 5 in, 1 out]
        n104 = Open VI Reference(vi path=w146, error in (no error)=w163) -> (vi reference=w160:refnum<vi>, error out=w159:errorcluster)  [unwired: 4 in]
        n105 = invoke on="Button Preview" class="SubPnl" method="Insert VI"(error in=w159, "VI Ref"=w160) -> (error out=w158:errorcluster)  [unwired: 2 in, 3 out]
        n106 = invoke class="VI" method="Run VI"(reference=w160, error in=w158, "Wait until done"=w168, "Auto Dispose Ref"=w168) -> (reference out=w143:refnum<vi>, error out=w156:errorcluster)  [unwired: 1 in, 3 out]
        n107 = Bundle By Name(cluster=w145, "subpanel VI ref"=w143) -> (w144:refnum<class "TSC Button Editor.lvclass">)
      }
      event User Event {
        w201 = FALSE ("Wait Until Done")
        # "run and reinsert the VI"
        # "abort to make the change"
        n108 = event-data() -> ()  [unwired: 1 in, 1 out]
        n109 = property on="Button Family" class="Ring (strict)"() -> ("RingText.Text"=w179:string)  [unwired: 2 in, 2 out]
        n110 = Unbundle By Name(w174) -> ("subpanel VI path"=w175:path, "Editor Theme"=w176:refnum<class "Material Theme.lvclass">, "subpanel VI ref"=w177:refnum<vi>)
        n111 = case shown="\"(3) Large Button Single Image 40px\", \"(6) Large Button Multi Image 40px\"" w179 {
          tunnel: [path "../assets/images/add_reaction.png" path "../assets/images/add_reaction_big.png"] -> w178
          frame Default {
          }
          frame "(3) Large Button Single Image 40px", "(6) Large Button Multi Image 40px" {
          }
        }
        n112 = invoke on="Button Preview" class="SubPnl" method="Remove VI"() -> (error out=w194:errorcluster)  [unwired: 3 in, 2 out]
        n113 = local read "Theme"() -> (w200:u16)
        n114 = invoke class="VI" method="Abort VI"(reference=w177, error in=w194) -> (reference out=w198:refnum<vi>, error out=w202:errorcluster)  [unwired: 1 in, 1 out]
        n115 = call "Get Scheme.vi"("Theme"=w200, "Material Theme in"=w176) -> ("Material-Scheme"=w195:refnum<class "Material-Scheme.lvclass">)  [unwired: 7 in, 2 out]
        n116 = Close Reference(reference=w198, error in (no error)=w202) -> (error out=w199:errorcluster)
        n117 = Cluster To Array(cluster="Multiple Colors") -> (array=w180:u32[])
        n118 = Cluster To Array(cluster="Button Images") -> (array=w182:path[])
        n119 = call <vilib>:"Clear Errors.vi"("error in (no error)"=w199) -> ("error out"=w197:errorcluster)  [unwired: 5 in, 1 out]
        n120 = Current VI's Path() -> (path=w189:path)
        n121 = Build Path(base path=w189, name or relative path=w178) -> (appended path=w188:path)
        n122 = for {
          N: 4 -> [_]
          tunnel: w188 -> [w212]
          tunnel: [w211] -> w187 mode=indexing
          tunnel: w182 -> [w210]
          i -> [w208]
          n123 = Index Array(array=w210, index=w208) -> (element=w209:path)
          n124 = Empty String/Path?(string/path=w209) -> (empty?=w213:bool)
          n125 = Select(t=w212, s=w213, f=w209) -> (s? t:f=w211:path)
        }
        n126 = for {
          N: 4 -> [_]
          tunnel: [w206] -> w184 mode=indexing
          tunnel: w180 -> [w205]
          i -> [w207]
          n127 = Index Array(array=w205, index=w207) -> (element=w206:u32)
        }
        n128 = call "Update Image (Multiple).vi"("Replace Image"=w187, "error in"=w197, "New Color"=w184, "New Control"=w175, "Material-Scheme.lvclass"=w195) -> ("error out"=w196:errorcluster)  [unwired: 4 in, 2 out]
        n129 = Open VI Reference(vi path=w175, error in (no error)=w196) -> (vi reference=w193:refnum<vi>, error out=w192:errorcluster)  [unwired: 4 in]
        n130 = invoke on="Button Preview" class="SubPnl" method="Insert VI"(error in=w192, "VI Ref"=w193) -> (error out=w191:errorcluster)  [unwired: 2 in, 3 out]
        n131 = invoke class="VI" method="Run VI"(reference=w193, error in=w191, "Wait until done"=w201, "Auto Dispose Ref"=w201) -> (reference out=w172:refnum<vi>, error out=w190:errorcluster)  [unwired: 1 in, 3 out]
        n132 = Bundle By Name(cluster=w174, "subpanel VI ref"=w172) -> (w173:refnum<class "TSC Button Editor.lvclass">)
      }
      event "update colors", "Boolean Colors": Value Change {
        w221 = refnum<vi> refnum  # Boolean
        n133 = event-data() -> ()  [unwired: 1 in, 1 out]
        n134 = Unbundle By Name(w217) -> ("subpanel VI ref"=w215:refnum<vi>)
        n135 = Unbundle By Name("Boolean Colors") -> ("false color"=w229:cluster{"border":u32, "fill":u32}, "true color"=w228:cluster{"border":u32, "fill":u32}, "click true color"=w223:cluster{"border":u32, "fill":u32}, "click false color"=w224:cluster{"border":u32, "fill":u32}, "hover false color"=w227:cluster{"border":u32, "fill":u32}, "hover true color"=w226:cluster{"border":u32, "fill":u32})
        n136 = property class="VI"(reference=w215) -> ("Panel"=w234:refnum<vi>)  [unwired: 1 in, 2 out]
        n137 = property class="Pnl"(reference=w234) -> (error out=w232:errorcluster, "Controls[]"=w219:refnum<vi>[])  [unwired: 1 in, 1 out]
        n138 = Build Array(w229, w228, w223, w224, w227, w226) -> (w225:cluster{"border":u32, "fill":u32}[])
        n139 = Index Array(array=w219) -> (element=w218:refnum<vi>)  [unwired: 1 in]
        n140 = To More Specific Class(target class=w221, reference=w218, error in=w232) -> (specific class reference=w222:refnum<vi>, error out=w220:errorcluster)
        n141 = property class="Bool"(reference=w222, error in=w220, "Colors [4]"=w225) -> (error out=w233:errorcluster)  [unwired: 1 out]
        n142 = invoke class="VI" method="Save.Instrument"(reference=w215, error in=w233) -> (reference out=w214:refnum<vi>, error out=w231:errorcluster)  [unwired: 4 in, 4 out]
        n143 = Bundle By Name(cluster=w217, "subpanel VI ref"=w214) -> (w216:refnum<class "TSC Button Editor.lvclass">)
      }
      event "Boolean Text": Value Change {
        w241 = refnum<vi> refnum  # Boolean
        n144 = event-data() -> ()  [unwired: 1 in, 1 out]
        n145 = Unbundle By Name(w236) -> ("subpanel VI ref"=w238:refnum<vi>)
        n146 = property class="VI"(reference=w238) -> ("Panel"=w248:refnum<vi>)  [unwired: 1 in, 2 out]
        n147 = property class="Pnl"(reference=w248) -> (error out=w245:errorcluster, "Controls[]"=w247:refnum<vi>[])  [unwired: 1 in, 1 out]
        n148 = Index Array(array=w247) -> (element=w239:refnum<vi>)  [unwired: 1 in]
        n149 = To More Specific Class(target class=w241, reference=w239, error in=w245) -> (specific class reference=w242:refnum<vi>, error out=w240:errorcluster)
        n150 = property class="Bool"(reference=w242, error in=w240, "BoolText.Text"="Boolean Text") -> (error out=w246:errorcluster)  [unwired: 1 out]
        n151 = invoke class="VI" method="Save.Instrument"(reference=w238, error in=w246) -> (reference out=w237:refnum<vi>, error out=w243:errorcluster)  [unwired: 4 in, 4 out]
        n152 = Bundle By Name(cluster=w236, "subpanel VI ref"=w237) -> (w235:refnum<class "TSC Button Editor.lvclass">)
      }
      event "Button Size", "update button size": Value Change {
        w258 = refnum<vi> refnum  # Boolean
        n153 = event-data() -> ()  [unwired: 1 in, 1 out]
        n154 = Unbundle By Name(w250) -> ("subpanel VI ref"=w252:refnum<vi>)
        n155 = property class="VI"(reference=w252) -> ("Panel"=w261:refnum<vi>)  [unwired: 1 in, 2 out]
        n156 = property class="Pnl"(reference=w261) -> ("Controls[]"=w257:refnum<vi>[])  [unwired: 1 in, 2 out]
        n157 = Index Array(array=w257) -> (element=w260:refnum<vi>)  [unwired: 1 in]
        n158 = To More Specific Class(target class=w258, reference=w260) -> (specific class reference=w259:refnum<vi>, error out=w255:errorcluster)  [unwired: 1 in]
        n159 = property class="Bool"(reference=w259, error in=w255, "Button Size"="Button Size") -> (error out=w254:errorcluster)  [unwired: 1 out]
        n160 = invoke class="VI" method="Save.Instrument"(reference=w252, error in=w254) -> (reference out=w251:refnum<vi>, error out=w253:errorcluster)  [unwired: 4 in, 4 out]
        n161 = Bundle By Name(cluster=w250, "subpanel VI ref"=w251) -> (w249:refnum<class "TSC Button Editor.lvclass">)
      }
      event "update button text location", "Button Text Location": Value Change {
        w272 = refnum<vi> refnum  # Boolean
        n162 = event-data() -> ()  [unwired: 1 in, 1 out]
        n163 = Unbundle By Name(w265) -> ("subpanel VI ref"=w266:refnum<vi>)
        n164 = property class="VI"(reference=w266) -> ("Panel"=w275:refnum<vi>)  [unwired: 1 in, 2 out]
        n165 = property class="Pnl"(reference=w275) -> ("Controls[]"=w271:refnum<vi>[])  [unwired: 1 in, 2 out]
        n166 = Index Array(array=w271) -> (element=w274:refnum<vi>)  [unwired: 1 in]
        n167 = To More Specific Class(target class=w272, reference=w274) -> (specific class reference=w273:refnum<vi>)  [unwired: 1 in, 1 out]
        n168 = Add(x="Button Text Location", y=cluster{"Left":i32, "Top":i32} {"Left"=24, "Top"=36}) -> (x+y=w269:cluster{"Left":i32, "Top":i32})
        n169 = property class="Bool"(reference=w273, "BoolText.Position"=w269) -> (error out=w263:errorcluster)  [unwired: 1 in, 1 out]
        n170 = invoke class="VI" method="Save.Instrument"(reference=w266, error in=w263) -> (reference out=w267:refnum<vi>, error out=w262:errorcluster)  [unwired: 4 in, 4 out]
        n171 = Bundle By Name(cluster=w265, "subpanel VI ref"=w267) -> (w264:refnum<class "TSC Button Editor.lvclass">)
      }
      event "Lock Text in Center?": Value Change {
        w287 = refnum<vi> refnum  # Boolean
        n172 = event-data() -> ()  [unwired: 1 in, 1 out]
        n173 = Unbundle By Name(w277) -> ("subpanel VI ref"=w276:refnum<vi>)
        n174 = property class="VI"(reference=w276) -> ("Panel"=w290:refnum<vi>)  [unwired: 1 in, 2 out]
        n175 = property class="Pnl"(reference=w290) -> ("Controls[]"=w286:refnum<vi>[])  [unwired: 1 in, 2 out]
        n176 = Index Array(array=w286) -> (element=w289:refnum<vi>)  [unwired: 1 in]
        n177 = To More Specific Class(target class=w287, reference=w289) -> (specific class reference=w288:refnum<vi>)  [unwired: 1 in, 1 out]
        n178 = property class="Bool"(reference=w288, "LockBoolText"="Lock Text in Center?") -> (error out=w280:errorcluster, "BoolText.Position"=w282:T8)  [unwired: 1 in, 1 out]
        n179 = Subtract(x=w282, y=cluster{"Left":i32, "Top":i32} {"Left"=24, "Top"=36}) -> (x-y=w284:T8)
        n180 = local write "Button Text Location"(w284) -> ()
        n181 = invoke class="VI" method="Save.Instrument"(error in=w280) -> (reference out=w281:refnum<vi>, error out=w279:errorcluster)  [unwired: 5 in, 4 out]
        n182 = Bundle By Name(cluster=w277, "subpanel VI ref"=w281) -> (w278:refnum<class "TSC Button Editor.lvclass">)
      }
      event "Boolean Text Format", "update text format": Value Change {
        w300 = refnum<vi> refnum  # Boolean
        n183 = event-data() -> ()  [unwired: 1 in, 1 out]
        n184 = Unbundle By Name(w292) -> ("subpanel VI ref"=w291:refnum<vi>)
        n185 = property class="VI"(reference=w291) -> ("Panel"=w308:refnum<vi>)  [unwired: 1 in, 2 out]
        n186 = Unbundle By Name("Boolean Text Format") -> ("Font:Color"=w305:u32, "Font:Bold?"=w304:bool, "Font:Name"=w303:string, "Font:Size"=w302:u32)
        n187 = property class="Pnl"(reference=w308) -> (error out=w307:errorcluster, "Controls[]"=w298:refnum<vi>[])  [unwired: 1 in, 1 out]
        n188 = Index Array(array=w298) -> (element=w297:refnum<vi>)  [unwired: 1 in]
        n189 = To More Specific Class(target class=w300, reference=w297, error in=w307) -> (specific class reference=w301:refnum<vi>, error out=w299:errorcluster)
        n190 = property class="Bool"(reference=w301, error in=w299, "BoolText.FontColor"=w305, "BoolText.TextColor"=w305, "BoolText.FontBold"=w304, "BoolText.FontName"=w303, "BoolText.FontSize"=w302) -> (error out=w295:errorcluster)  [unwired: 1 out]
        n191 = invoke class="VI" method="Save.Instrument"(error in=w295) -> (reference out=w296:refnum<vi>, error out=w294:errorcluster)  [unwired: 5 in, 4 out]
        n192 = Bundle By Name(cluster=w292, "subpanel VI ref"=w296) -> (w293:refnum<class "TSC Button Editor.lvclass">)
      }
      event "Save": Value Change {
        n193 = event-data() -> ()  [unwired: 1 in, 1 out]
        n194 = Unbundle By Name(w310) -> ("subpanel VI ref"=w309:refnum<vi>)
        n195 = call "File Dialog"("pattern (all files)"="*.ctl" ("pattern label")) -> ("selected path"=w312:path, "error out"=w313:errorcluster)  [unwired: 11 in, 2 out]
        n196 = property class="VI"(reference=w309) -> ("Panel"=w317:refnum<vi>)  [unwired: 1 in, 2 out]
        n197 = property class="Pnl"(reference=w317) -> ("Controls[]"=w316:refnum<vi>[])  [unwired: 1 in, 2 out]
        n198 = Index Array(array=w316) -> (element=w315:refnum<vi>)  [unwired: 1 in]
        n199 = case shown="No Error" w313 {
          selector: w313 -> [w328 w338]
          tunnel: w315 -> [w333 _]
          tunnel: [w330 w337] -> w314
          tunnel: w312 -> [w327 _]
          frame No Error {
            w322 = TRUE  # Is Persistent?
            # "#fix the control-level meta data tag"
            # "save as a .ctl file with the tag data applied for the control-level"
            n200 = New VI(8:w328, 9:T9."Control VI" ("vi type (standard vi)")) -> (0:w335:errorcluster, 3:w334:refnum<vi>)  [unwired: 5 in]
            n201 = invoke class="VI" method="Create from Reference"(reference=w334, error in=w335, "Source Object Ref"=w333) -> (reference out=w324:refnum<vi>, error out=w332:errorcluster, "New Object Ref"=w326:refnum<vi>)  [unwired: 4 in, 4 out]
            n202 = property on="Color Level" class="Ring (strict)"() -> ("RingText.Text"=w318:string)  [unwired: 2 in, 2 out]
            n203 = property class="Ctl"(reference=w326, error in=w332, "Position"=T8 {"Left"=24, "Top"=24}) -> (reference out=w320:refnum<vi>, error out=w321:errorcluster)
            n204 = invoke class="Ctl" method="Tag.Set Tag"(reference=w320, error in=w321, "TagName"="control-level" ("Tag Name"), "Value"=w318, "isPersistent"=w322) -> (error out=w319:errorcluster)  [unwired: 2 in, 6 out]
            n205 = invoke class="VI" method="Save.Instrument"(reference=w324, error in=w319, "Path to saved file"=w327) -> (reference out=w329:refnum<vi>, error out=w331:errorcluster)  [unwired: 3 in, 4 out]
            n206 = Close Reference(reference=w329, error in (no error)=w331) -> (error out=w330:errorcluster)
          }
          frame Error {
            n207 = Unbundle By Name(w338) -> ("code"=w339:i32)
            n208 = case shown="Default" w339 {
              tunnel: w338 -> [_ w340]
              tunnel: [_ w340] -> w337
              frame 43 {
              }
              frame Default {
              }
            }
          }
        }
      }
      event Menu Selection (User) {
        n209 = event-data() -> ("ItemTag"=w343:string)  [unwired: 1 in]
        n210 = Unbundle By Name(w342) -> ("subpanel VI ref"=w341:refnum<vi>)
        n211 = case shown="\"save\"" w343 {
          tunnel: w341 -> [_ w351]
          tunnel: [_ w348] -> w344
          frame Default {
          }
          frame "save" {
            # "Ctrl+S menu shortcut"
            n212 = call "File Dialog3"("pattern (all files)"="*.ctl" ("pattern label")) -> ("selected path"=w346:path, "error out"=w347:errorcluster)  [unwired: 11 in, 2 out]
            n213 = property class="VI"(reference=w351) -> ("Panel"=w352:refnum<vi>)  [unwired: 1 in, 2 out]
            n214 = property class="Pnl"(reference=w352) -> ("Controls[]"=w350:refnum<vi>[])  [unwired: 1 in, 2 out]
            n215 = Index Array(array=w350) -> (element=w349:refnum<vi>)  [unwired: 1 in]
            n216 = case shown="No Error" w347 {
              selector: w347 -> [w363 w373]
              tunnel: w349 -> [w368 _]
              tunnel: [w365 w372] -> w348
              tunnel: w346 -> [w362 _]
              frame No Error {
                # "#fix the control-level meta data tag"
                n217 = New VI(8:w363, 9:T9."Control VI" ("vi type (standard vi)")) -> (0:w370:errorcluster, 3:w369:refnum<vi>)  [unwired: 5 in]
                n218 = invoke class="VI" method="Create from Reference"(reference=w369, error in=w370, "Source Object Ref"=w368) -> (reference out=w359:refnum<vi>, error out=w367:errorcluster, "New Object Ref"=w361:refnum<vi>)  [unwired: 4 in, 4 out]
                n219 = property on="Color Level" class="Ring (strict)"() -> ("RingText.Text"=w358:string)  [unwired: 2 in, 2 out]
                n220 = property class="Ctl"(reference=w361, error in=w367, "Position"=T8 {"Left"=24, "Top"=24}) -> (reference out=w354:refnum<vi>, error out=w355:errorcluster)
                n221 = invoke class="Ctl" method="Tag.Set Tag"(reference=w354, error in=w355, "TagName"="control-level" ("Tag Name"), "Value"=w358, "isPersistent"=TRUE ("Is Persistent?")) -> (error out=w353:errorcluster)  [unwired: 2 in, 6 out]
                n222 = invoke class="VI" method="Save.Instrument"(reference=w359, error in=w353, "Path to saved file"=w362) -> (reference out=w364:refnum<vi>, error out=w366:errorcluster)  [unwired: 3 in, 4 out]
                n223 = Close Reference(reference=w364, error in (no error)=w366) -> (error out=w365:errorcluster)
              }
              frame Error {
                n224 = Unbundle By Name(w373) -> ("code"=w374:i32)
                n225 = case shown="43" w374 {
                  tunnel: w373 -> [_ w375]
                  tunnel: [_ w375] -> w372
                  frame 43 {
                  }
                  frame Default {
                  }
                }
              }
            }
          }
        }
      }
      event "Button Type": Value Change {
        w402 = FALSE ("Wait Until Done")
        # "rerun and reinsert VI with new control"
        # "open the selected ctl and replace old one"
        # "abort and remove temporarily"
        n226 = event-data() -> ()  [unwired: 1 in, 1 out]
        n227 = Unbundle By Name(w380) -> ("subpanel VI path"=w381:path, "subpanel VI ref"=w377:refnum<vi>, "control top level"=w376:path)
        n228 = Unbundle By Name(w390) -> ("update colors"=w389:refnum<user-event>)
        n229 = invoke class="VI" method="Abort VI"(reference=w377) -> (error out=w395:errorcluster)  [unwired: 2 in, 2 out]
        n230 = property on="Button Family" class="Ring (strict)"() -> ("RingText.Text"=w385:string)  [unwired: 2 in, 2 out]
        n231 = Generate User Event(user event=w389, event data cluster=variant ("event data")) -> ()  [unwired: 2 in, 2 out]
        n232 = invoke on="Button Preview" class="SubPnl" method="Remove VI"(error in=w395) -> (error out=w394:errorcluster)  [unwired: 2 in, 2 out]
        n233 = Build Path(base path=w376, name or relative path=w385) -> (appended path=w386:path)
        n234 = call <vilib>:"Clear Errors.vi"("error in (no error)"=w394) -> ("error out"=w393:errorcluster)  [unwired: 5 in, 1 out]
        n235 = property class="VI"(reference=w377, error in=w393) -> (reference out=w391:refnum<vi>, error out=w398:errorcluster, "Panel"=w412:refnum<vi>)
        n236 = List Folder(path=w386, pattern="*.ctl") -> (path out=w408:path, filenames=w409:string[])  [unwired: 2 in, 2 out]
        n237 = property class="Pnl"(reference=w412, error in=w398) -> (error out=w397:errorcluster, "Controls[]"=w411:refnum<vi>[])  [unwired: 1 out]
        n238 = Index Array "Index Array"(array=w409, index="Button Type") -> (element=w407:string)
        n239 = Index Array(array=w411) -> (element=w406:refnum<vi>)  [unwired: 1 in]
        n240 = Build Path(base path=w408, name or relative path=w407) -> (appended path=w387:path)
        n241 = invoke class="Ctl" method="Replace No Attrib"(reference=w406, error in=w397, "Param 1"=w387) -> (error out=w399:errorcluster, "RepNoAttrib"=w382:refnum<vi>)  [unwired: 3 in, 4 out]
        n242 = property class="GObj"(reference=w382, error in=w399, "Position"=T8 {"Left"=0, "Top"=0}) -> (error out=w384:errorcluster)  [unwired: 1 out]
        n243 = invoke class="VI" method="Save.Instrument"(reference=w391, error in=w384) -> (error out=w392:errorcluster)  [unwired: 4 in, 5 out]
        n244 = Close Reference(reference=w391, error in (no error)=w392) -> (error out=w400:errorcluster)
        n245 = Open VI Reference(vi path=w381, error in (no error)=w400) -> (vi reference=w403:refnum<vi>, error out=w404:errorcluster)  [unwired: 4 in]
        n246 = invoke class="VI" method="Run VI"(reference=w403, error in=w404, "Wait until done"=w402, "Auto Dispose Ref"=w402) -> (reference out=w378:refnum<vi>, error out=w396:errorcluster)  [unwired: 1 in, 3 out]
        n247 = Bundle By Name(cluster=w380, "subpanel VI ref"=w378) -> (w379:refnum<class "TSC Button Editor.lvclass">)
        n248 = invoke on="Button Preview" class="SubPnl" method="Insert VI"(error in=w396, "VI Ref"=w378) -> (error out=w401:errorcluster)  [unwired: 2 in, 3 out]
      }
      event "Button Family": Value Change {
        w417 = u16 0 items=[""] ("Button Type")
        n249 = event-data() -> ()  [unwired: 1 in, 1 out]
        n250 = property on="Button Family" class="Ring (strict)"() -> ("RingText.Text"=w415:string)  [unwired: 2 in, 2 out]
        n251 = Unbundle By Name(w414) -> ("control top level"=w413:path)
        n252 = case shown="\"(2) Small Button Text Only\", \"(4) Large Button Text Only\"" w415 {
          tunnel: [TRUE FALSE FALSE] -> w421
          tunnel: [FALSE TRUE FALSE] -> w420
          frame Default {
          }
          frame "(5) Small Button Multi Image 24px", "(6) Large Button Multi Image 40px" {
          }
          frame "(2) Small Button Text Only", "(4) Large Button Text Only" {
          }
        }
        n253 = property on="Button Image" class="Path"("Visible"=w421) -> ()  [unwired: 2 in, 2 out]
        n254 = property on="Button Images" class="Clust (strict)"("Visible"=w420) -> ()  [unwired: 2 in, 2 out]
        n255 = property on="Image Color" class="ColBox"("Visible"=w421) -> ()  [unwired: 2 in, 2 out]
        n256 = property on="Multiple Colors" class="Clust (strict)"("Visible"=w420) -> ()  [unwired: 2 in, 2 out]
        n257 = Build Path(base path=w413, name or relative path=w415) -> (appended path=w419:path)
        n258 = List Folder(path=w419, pattern="*.ctl") -> (filenames=w416:string[])  [unwired: 2 in, 3 out]
        n259 = property on="Button Type" class="Ring (strict)"("Strings []"=w416, "Val(Sgnl)"=w417) -> ()  [unwired: 2 in, 2 out]
      }
      event "Open": Value Change {
        n260 = event-data() -> ()  [unwired: 1 in, 1 out]
        n261 = call "File Dialog2"("pattern label"="*.ctl") -> ("selected path"=w429:path, "error out"=w431:errorcluster)  [unwired: 11 in, 2 out]
        n262 = case shown="No Error" w431 {
          selector: w431 -> [_ w488]
          tunnel: [w439 w487] -> w430
          tunnel: w429 -> [w444 _]
          tunnel: w428 -> [w435 _]
          frame No Error {
            w441 = FALSE ("Wait Until Done")
            w480 = refnum<vi> refnum  # Boolean
            # "#update \nNeeds:\n-pull out the meta-data for the control level and button type\n-how the heck do i figure out the theme file it was saved with?? - add other tag?? hmmm........\n-need color of image also"
            n263 = Unbundle By Name(w435) -> ("subpanel VI path"=w433:path, "subpanel VI ref"=w434:refnum<vi>)
            n264 = invoke on="Button Preview" class="SubPnl" method="Remove VI"() -> (error out=w443:errorcluster)  [unwired: 3 in, 2 out]
            n265 = invoke class="VI" method="Abort VI"(reference=w434, error in=w443) -> (reference out=w449:refnum<vi>, error out=w460:errorcluster)  [unwired: 1 in, 1 out]
            n266 = Close Reference(reference=w449, error in (no error)=w460) -> (error out=w454:errorcluster)
            n267 = call <vilib>:"Clear Errors.vi"("error in (no error)"=w454) -> ("error out"=w453:errorcluster)  [unwired: 5 in, 1 out]
            n268 = Open VI Reference(vi path=w444, error in (no error)=w453) -> (vi reference=w450:refnum<vi>, error out=w451:errorcluster)  [unwired: 4 in]
            n269 = property class="VI"(reference=w450, error in=w451) -> (reference out=w445:refnum<vi>, error out=w479:errorcluster, "Panel"=w481:refnum<vi>)
            n270 = property class="Pnl"(reference=w481, error in=w479) -> (error out=w478:errorcluster, "Controls[]"=w484:refnum<vi>[])  [unwired: 1 out]
            n271 = Index Array(array=w484) -> (element=w482:refnum<vi>)  [unwired: 1 in]
            n272 = To More Specific Class(target class=w480, reference=w482, error in=w478) -> (specific class reference=w483:refnum<vi>, error out=w459:errorcluster)
            n273 = property class="Bool"(reference=w483, error in=w459) -> (error out=w448:errorcluster, "Position"=w455:T8, "Label.Height"=w456:u32, "Button Size"=w477:T10, "BoolText.Text"=w476:string, "BoolText.TextColor"=w475:u32, "BoolText.FontBold"=w474:bool, "BoolText.FontName"=w473:string, "BoolText.FontSize"=w472:u32, "Colors [4]"=w467:cluster{u32, u32}[])  [unwired: 1 out]
            n274 = Close Reference(reference=w445, error in (no error)=w448) -> (error out=w446:errorcluster)
            n275 = Index Array(array=w467) -> (element #1=w466:cluster{u32, u32}, element #2=w465:cluster{u32, u32}, element #3=w464:cluster{u32, u32}, element #4=w463:cluster{u32, u32}, element #5=w462:cluster{u32, u32}, element #6=w461:cluster{u32, u32})  [unwired: 6 in]
            n276 = Open VI Reference(vi path=w433, error in (no error)=w446) -> (vi reference=w437:refnum<vi>, error out=w447:errorcluster)  [unwired: 4 in]
            n277 = Bundle By Name(cluster=T1 {"false color"={"border"=15922170, "fill"=15922170}, "true color"={"border"=14936305, "fill"=14936305}, "click false color"={"border"=14410221, "fill"=14410221}, "click true color"={"border"=14410221, "fill"=14410221}, "hover false color"={"border"=14540516, "fill"=14540516}, "hover true color"={"border"=14540516, "fill"=14540516}} ("Boolean Colors"), "false color"=w466, "true color"=w465, "click true color"=w464, "click false color"=w463, "hover false color"=w462, "hover true color"=w461) -> (w468:T1)
            n278 = call "Update Custom UI for Button.vi"("error in"=w447, "selected path"=w444, "vi reference"=w437) -> ("error out"=w440:errorcluster, "appended path"=w438:path, "vi reference out"=w436:refnum<vi>)  [unwired: 6 in]
            n279 = invoke on="Button Preview" class="SubPnl" method="Insert VI"(error in=w440, "VI Ref"=w436) -> (error out=w442:errorcluster)  [unwired: 2 in, 3 out]
            n280 = Bundle By Name(cluster=T2 {"Font:Color"=3563918, "Font:Bold?"=TRUE, "Font:Name"="App Font", "Font:Size"=22} ("Boolean Text Format"), "Font:Color"=w475, "Font:Bold?"=w474, "Font:Name"=w473, "Font:Size"=w472) -> (w471:T2)
            n281 = local write "Boolean Colors"(w468) -> ()
            n282 = invoke class="VI" method="Run VI"(reference=w436, error in=w442, "Wait until done"=w441, "Auto Dispose Ref"=w441) -> (error out=w439:errorcluster)  [unwired: 1 in, 4 out]
            n283 = Unbundle By Name(w455) -> ("Top"=w458:i32)
            n284 = local write "Boolean Text Format"(w471) -> ()
            n285 = Add(x=w458, y=w456) -> (x+y=w457:u32)
            n286 = Bundle By Name(cluster=w455, "Top"=w457) -> ()  [unwired: 1 out]
            n287 = flat-sequence {
              tunnel: w438 -> [w486]
              tunnel: [w485] -> w452
              tunnel: w439 -> [_]
              frame #0 {
                n288 = call "Read Image on Button.vi"("File with Button"=w486) -> ("png file out"=w485:path)  [unwired: 9 in, 1 out]
              }
            }
            n289 = local write "Button Size"(w477) -> ()
            n290 = local write "Boolean Text"(w476) -> ()
            n291 = local write "Button Image"(w452) -> ()
          }
          frame Error {
            n292 = Unbundle By Name(w488) -> ("code"=w489:i32)
            n293 = case shown="Default" w489 {
              tunnel: w488 -> [w490 _]
              tunnel: [w490 _] -> w487
              frame Default {
              }
              frame 43 {
              }
            }
          }
        }
      }
    }
    "error out" <- w34
    n294 = call <vilib>:"Simple Error Handler.vi"("error in (no error)"=w34) -> ()  [unwired: 4 in, 5 out]
  }
  n295 = call "User Event Close.vi"("Event Registration Refnum"=w25, "user events"=w24) -> ()  [unwired: 9 in, 1 out]
  n296 = flat-sequence {
    frame #0 {
      n297 = disable-structure shown="Disabled" {
        frame Disabled {
          n298 = control-ref of="This VI"() -> (w491:refnum<vi>)
          n299 = invoke class="VI" method="FP.Close"(reference=w491) -> ()  [unwired: 2 in, 3 out]
        }
        frame Enabled {
        }
      }
    }
  }
  n300 = Unbundle By Name(w7) -> ("subpanel VI ref"=w6:refnum<vi>)
  n301 = invoke class="VI" method="Abort VI"(reference=w6) -> (reference out=w30:refnum<vi>, error out=w29:errorcluster)  [unwired: 2 in, 1 out]
  n302 = Close Reference(reference=w30, error in (no error)=w29) -> ()  [unwired: 1 out]
